vi "Micro-PL v10.5.0.vi"() -> ()   [LabVIEW 2010]
uses:
  drivers/Oxford ITC/ITCAPPS.LLB/ITCSetup.ctl
  drivers/Oxford ITC/ITCSUBS.LLB/ITCIO.ctl
  drivers/Oxford ITC/BUSGEN.LLB/OxfordAddress.ctl
  drivers/Oxford ITC/ITCSUBS.LLB/ITCVersion.ctl
  subvi/ESA-C/TypeDefs/ESA-C Live Controls v10.4.0.ctl
  subvi/ESA-C/TypeDefs/ESA-C Current Values.ctl
  subvi/ESA-C/TypeDefs/ESA-C Connection Settings.ctl
  subvi/ESA-C/TypeDefs/ESA-C Set Positions.ctl
  subvi/ITC503/TypeDefs/ITC503 Settings.ctl
  subvi/ITC503/TypeDefs/ITC503 Current Values.ctl
  subvi/iHR550/TypeDefs/iHR Current Values.ctl
  subvi/iHR550/TypeDefs/iHR Settings.ctl
  subvi/Mapping/TypeDefs/Mapping Spectra Params.ctl
  <vilib>/Utility/miscctls.llb/LVBoundsTypeDef.ctl
  subvi/Symphony/TypeDefs/Symphony Area Format.ctl
  <vilib>/Utility/miscctls.llb/LVPointTypeDef.ctl
  subvi/Mapping/TypeDefs/Mapping Input Parameters.ctl
  subvi/Global Variables.vi
  <vilib>/Analysis/NI_AALBase.lvlib
panel:
  out "Spectrum Raw PX":dbl[][](array[numeric])
  out "Image Raw":i32[][](array[numeric])
  in  "Wavelength Recalculate":bool
  out "CCD Error":errorcluster
  out "Firmware":string="V1.20 CCD_4000"
  out "CCD Gain Number":i32[](array[numeric])=[10, 11, 12, 13, 8, 2]
  out "CCD ADC Number":i32[](array[numeric])=[0, 1, 2, 3, 4]
  out "JYCCDLib.IJYCCDReqd":refnum<k7>
  out "Spectrum Raw WL":dbl[][](array[numeric])
  out "Mapping State Storage":bool
  out "Drive Copy Target":bool
  in  "CCD Shutter":bool caption="Shutter:"
  out "Measurement Running":bool
  out "ITC Running":bool
  out "Drive Running":bool
  out "CCD Running":bool
  out "Mono Running":bool
  in  "Exit":bool
  out "Mono Status":bool
  out "Drive Status":bool
  out "CCD Status":bool
  out "ITC Status":bool
  in  "Register":enum32{"Devices", "Acquisition / Mapping"}(tab)
  in  "CCD Gain":u16(ring)=1 caption="Gain Mode" items=["High Light", "Best Dynamic Range", "High Sensitivity"]
  in  "Image Mode":bool caption="Image Mode?"
  in  "CCD Names":u16(ring) caption="CCD ID" items=["Symphony II"]
  in  "CCD Connect":bool
  out "CCD Temperature":dbl caption="Temp. (°C)" min=10.0 max=160.0 step=0.1 format="%.1f"
  out "CCD Pixel X":i32=2048 caption="X Pixels"
  out "CCD Pixel Y":i32=512 caption="Y Pixels"
  out "CCD Data Size":i32=2048 caption="Data Size"
  in  "CCD ADC":u16(ring) caption="ADC Frequency" items=["20 kHz       ", " 1 MHz       ", " 1 MHz Ultra ", "500 kHz Wrap"]
  in  "CCD Configure":bool
  in  "CCD Area":T1={"XStart"=1, "YStart"=1, "XStop"=2048, "YStop"=512, "XBin"=1, "YBin"=1}
  in  "Snapshot Folder":path=path "C:/Users/WET-KORR/Desktop/Screenshots"
  in  "Camera Name":string="HD USB Camera"
  out "CCD Temp Graph":dbl(graph)=-134.538067
  out "CCD IDs":u16(ring) items=["CCD1"]
  out "ITC Current Values":T2 {"ITC503 Gradient" format="%.2f"; "ITC503 Setpoint" min=-273.0 max=300000.0 step=0.0001 format="%.1f"; "ITC503 I" format="%_1f"; "ITC503 P" format="%_1f"; "ITC503 Temperature" min=0.0 max=1645.0 step=1e-05 format="%.2f"; "ITC503 Heater" min=0.0 max=100.0 step=0.01 scale=0.0..100.0}
  in  "ITC Settings":T3={"ITC503 Set Setpoint"=0.0, "ITC503 Set Auto Heater"=TRUE, "ITC503 Set Auto PID"=TRUE, "P"=0.0, "I"=0.0, "D"=0.0} {"D" min=0.0 max=100.0 step=0.1 format="%.1f"; "I" min=0.0 max=100.0 step=0.1 format="%.1f"; "P" min=0.0 max=100.0 step=0.1 format="%.1f"; "ITC503 Set Setpoint" min=-273.0 max=300000.0 step=0.1 format="%.1f"}
  in  "ITC Configure":bool
  in  "ITC Connect":bool
  in  "ITC Selector":u16(ring) caption="Select Device" items=["ITC503s"]
  out "Drive Current Values":T4 {"Position"."Drive Z Position" min=-273.0 max=300000.0 step=0.0001 format="%.1f"; "Position"."Drive Y Position" min=-273.0 max=300000.0 step=0.0001 format="%.1f"; "Position"."Drive X Position" min=-273.0 max=300000.0 step=0.0001 format="%.1f"; "Voltages"."Drive Z Voltage" min=-273.0 max=300000.0 step=0.0001 format="%.1f"; "Voltages"."Drive Y Voltage" min=-273.0 max=300000.0 step=0.0001 format="%.1f"; "Voltages"."Drive X Voltage" min=-273.0 max=300000.0 step=0.0001 format="%.1f"}
  in  "Drive Connection":T5={"Objective GPIB-Port"=4, "Stage GPIB-Port"=4, "Drive Selector"=0, "Drive Velocity (V/s)"=5.0} {"Drive Velocity (V/s)" min=10.0 max=160.0 step=0.1 format="%.1f"; "Drive Selector" items=["Obj.", "Stage"]; "Stage GPIB-Port" min=1 max=20 step=1 format="%#.0f"; "Objective GPIB-Port" min=1 max=20 step=1 format="%#.0f"}
  in  "Drive Connect":bool
  in  "Mono Force Init":bool=TRUE caption="iHR550 Force Init"
  in  "Mono Connect":bool
  in  "Mono ID":string(combo)="iHR550" caption="Monochromator ID"
  out "Mono Timing":u32 caption="Mono"
  out "Drive Timing":u32 caption="Drive"
  out "ITC Timing":u32 caption="ITC"
  out "CCD Timing":u32 caption="CCD"
  in  "Spectrum Axis":u16(ring)=1 caption="Axis" items=["Pixel", "Wavelength", "Energy"]
  in  "Spectrum Autosave":bool caption="iHR550 Force Init"
  in  "CCD Preview":bool
  in  "CCD Acquire":bool
  in  "Spectrum Settings":T6={"Integration Time"=1.0, "Repetitions"=1, "Mapping Spectra"=TRUE} caption="Mapping Spectra Settings" {"Repetitions" min=1 max=100 step=1; "Integration Time" min=0.1 max=6000.0 step=0.1 format="%.1f"}
  in  "CCD Current Rep.":string="0/0"
  out "Spectrum":cluster{dbl[], dbl[]}[](graph)
  out "Image":dbl[][](graph)
  in  "Spectrum Noise":i64 caption="Noise Level"
  in  "Spectrum Load":bool
  in  "Spectrum Save":bool
  in  "Spectrum Maximize":bool
  in  "Video Show":bool
  in  "Drive GoTo":bool caption="Objective Move Abs."
  in  "Drive New Positions":T7 {"Drive X Set" min=10.0 max=160.0 step=0.1 format="%.1f"; "Drive Z Set" min=10.0 max=160.0 step=0.1 format="%.1f"; "Drive Y Set" min=10.0 max=160.0 step=0.1 format="%.1f"}
  in  "Mapping Start":bool
  in  "Mono Configure":bool
  in  "Mono Settings":T8={"iHR550 Set Exit Mirror"=2, "iHR550 Set Side Exit"=0.0, "iHR550 Set Front Entrance"=0.0, "iHR550 Set Wavelength"=897.9988, "iHR550 Set Grating"=0, "iHR550 Set Grating Switch"=FALSE, "iHR550 Set Wavelength Switch"=FALSE, "iHR550 Set Mirror Switch"=FALSE, "iHR550 Set Slits Switch"=FALSE} {"iHR550 Set Grating" items=["1800"=1, "600"=2, "150"=3]; "iHR550 Set Wavelength" min=0.0 max=1500.0 step=1.0; "iHR550 Set Side Exit" min=0.0 max=2000.0 step=1.0; "iHR550 Set Exit Mirror" items=["Front"=2, "Side"=3]}
  out "Mono Current Values":T9={"iHR 550 Front Entrance"=0.0, "iHR550 Side Exit"=0.0, "iHR550 Wavelength"=897.9988, "iHR550 Exit Mirror"=2, "iHR550 Grating"="1", "Grating Index"=1} {"iHR550 Exit Mirror" items=["EntranceMirror", "ExitMirror", "Front", "Side"]}
  out "Drive Live Current Values":T4 {"Position"."Drive Z Position" min=-273.0 max=300000.0 step=0.0001 format="%.1f"; "Position"."Drive Y Position" min=-273.0 max=300000.0 step=0.0001 format="%.1f"; "Position"."Drive X Position" min=-273.0 max=300000.0 step=0.0001 format="%.1f"; "Voltages"."Drive Z Voltage" min=-273.0 max=300000.0 step=0.0001 format="%.1f"; "Voltages"."Drive Y Voltage" min=-273.0 max=300000.0 step=0.0001 format="%.1f"; "Voltages"."Drive X Voltage" min=-273.0 max=300000.0 step=0.0001 format="%.1f"}
  in  "Drive Live Controls":T10={"Move Step"=1.0, "Move Home"=FALSE, "Move Down"=FALSE, "Move Up"=FALSE, "Move Left"=FALSE, "Move Right"=FALSE, "Move Out"=FALSE, "Move In"=FALSE} {"Move Step" min=0.0 max=30.0 step=0.1 format="%.1f"}
  out "ITC Temp Storage":dbl
  out "Runtime":u32
  out "ITC Gradient Time":i64
  out "ITC Read":bool
  out "CCD Read":bool
  out "Mono Read":bool
  out "Drive Read":bool
  out "Spectrum Properties":cluster{"Position":T11, "Plot Area Size":T11}={"Position"={"Width"=36, "Height"=367}, "Plot Area Size"={"Width"=496, "Height"=264}}
  in  "Auto Folder":path caption="Ausgewählter Pfad"
  out "Wavelengths (nm)":dbl[](array[numeric])
  out "iHR550 RefNum":refnum<k7> caption="Mono RefNum out"
  out "ITC Setup":T12={"Description"="", "IO Info"={"Address"={"Com Port"=1, "ISOBUS Address"=1, "GPIB Address"=24, "Communication"=enum."ISOBUS"}, "Version"=enum."ITC503", "Ch 1 dec places"=1, "Ch 2 dec places"=1, "Ch 3 dec places"=1, "Ch1 Name"="", "Ch2 Name"="", "Ch3 Name"=""}}
  # "Correlation Setup"
  # "Active"
  # "Active"
  # "ITC"
  # "iHR"
  # "Drive"
  # "CCD"
  # "Status"
  # "CCD"
  # "ITC"
  # "iHR"
  # "Drive"
  # "CCD"
  # "Video"
  # "Cryostat"
  # "Drives"
  # "Monochromator"
  # "Timing"
  # "Drive Control"
  # "CCD"
  # "Acquisition"
  # "Mapping"
  # "Launch the Spectral Mapping VI and Raman Tool Set 2.0 in a new window."
  # "Monochromator"
  # "XY"
  # "Z"
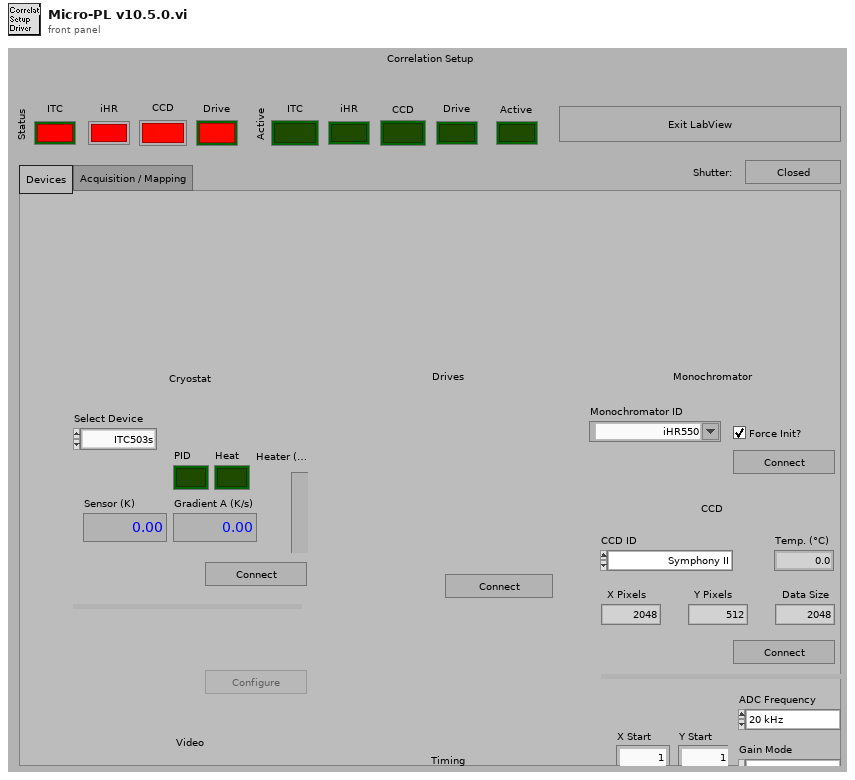
[diagram p1: front panel]
types:
  T1 = typedef "Symphony Area Format.ctl" = cluster{"XStart":i32, "YStart":i32, "XStop":i32, "YStop":i32, "XBin":i32, "YBin":i32}
  T2 = typedef "ITC503 Current Values.ctl" = cluster{"ITC503 Heater":dbl, "ITC503 Temperature":dbl, "ITC503 P":dbl, "ITC503 I":dbl, "ITC503 D":dbl, "ITC503 Setpoint":dbl, "ITC503 Gradient":dbl, "ITC503 Heater Auto":bool, "ITC503 PID Auto":bool}
  T3 = typedef "ITC503 Settings.ctl" = cluster{"ITC503 Set Setpoint":dbl, "ITC503 Set Auto Heater":bool, "ITC503 Set Auto PID":bool, "P":dbl, "I":dbl, "D":dbl}
  T4 = typedef "ESA-C Current Values.ctl" = cluster{"Voltages":cluster{"Drive X Voltage":dbl, "Drive Y Voltage":dbl, "Drive Z Voltage":dbl}, "Position":cluster{"Drive X Position":dbl, "Drive Y Position":dbl, "Drive Z Position":dbl}}
  T5 = typedef "ESA-C Connection Settings.ctl" = cluster{"Objective GPIB-Port":i32, "Stage GPIB-Port":i32, "Drive Selector":u16, "Drive Velocity (V/s)":dbl}
  T6 = typedef "Mapping Spectra Params.ctl" = cluster{"Integration Time":dbl, "Repetitions":u16, "Mapping Spectra":bool}
  T7 = typedef "ESA-C Set Positions.ctl" = cluster{"Drive X Set":dbl, "Drive Y Set":dbl, "Drive Z Set":dbl}
  T8 = typedef "iHR Settings.ctl" = cluster{"iHR550 Set Exit Mirror":u16, "iHR550 Set Side Exit":dbl, "iHR550 Set Front Entrance":dbl, "iHR550 Set Wavelength":dbl, "iHR550 Set Grating":u16, "iHR550 Set Grating Switch":bool, "iHR550 Set Wavelength Switch":bool, "iHR550 Set Mirror Switch":bool, "iHR550 Set Slits Switch":bool}
  T9 = typedef "iHR Current Values.ctl" = cluster{"iHR 550 Front Entrance":dbl, "iHR550 Side Exit":dbl, "iHR550 Wavelength":dbl, "iHR550 Exit Mirror":i32, "iHR550 Grating":string, "Grating Index":i32}
  T10 = typedef "ESA-C Live Controls v10.4.0.ctl" = cluster{"Move Step":dbl, "Move Home":bool, "Move Down":bool, "Move Up":bool, "Move Left":bool, "Move Right":bool, "Move Out":bool, "Move In":bool}
  T11 = typedef "LVBoundsTypeDef.ctl" = cluster{"Width":u32, "Height":u32}
  T12 = typedef "ITCSetup.ctl" = cluster{"Description":string, "IO Info":T13}
  T13 = typedef "ITCIO.ctl" = cluster{"Address":T14, "Version":T15, "Ch 1 dec places":i16, "Ch 2 dec places":i16, "Ch 3 dec places":i16, "Ch1 Name":string, "Ch2 Name":string, "Ch3 Name":string}
  T14 = typedef "OxfordAddress.ctl" = cluster{"Com Port":i32, "ISOBUS Address":i32, "GPIB Address":i16, "Communication":enum16{"RS232", "ISOBUS", "GPIB", "Gateway"}}
  T15 = typedef "ITCVersion.ctl" = enum16{"ITC502", "ITC503", "ITC601"}
  T16 = enum8{"Enabled", "Disabled", "Disabled and Grayed Out"}
  T17 = typedef "LVPointTypeDef.ctl" = cluster{"Horizontal":i16, "Vertical":i16}
  T18 = typedef "Mapping Input Parameters.ctl" = cluster{"Drive Connection Settings":T5, "ITC503 Current Values":T2, "Wavelengths (nm)":dbl[], "Drive Current Values":T4, "iHR Current Values":T9, "Spectra Settings":T6, "CCD3500 Temperature":dbl, "Simulate Drive":bool, "Simulate Spectra":bool, "JYCCDLib.IJYCCDReqd":refnum<k7>}
  T19 = cluster{"Intensities":dbl[], "Wavelengths":dbl[]}[]
  T20 = cluster{"Drive X Position":dbl, "Drive Y Position":dbl, "Drive Z Position":dbl}
  T21 = typedef "LVPositionTypeDef.ctl" = cluster{"Left":i32, "Top":i32}
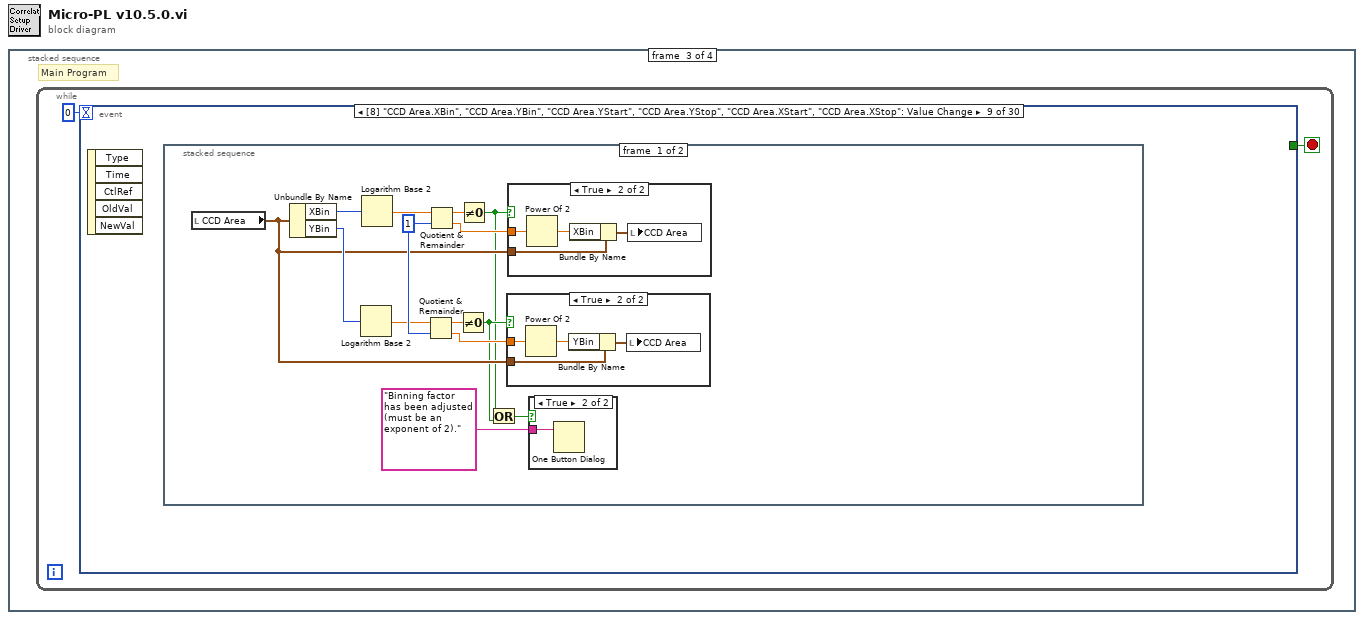
[diagram p0: block diagram]
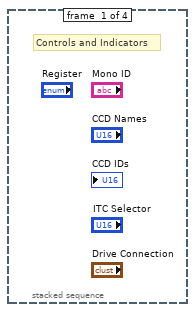
[diagram p2: hidden frame]
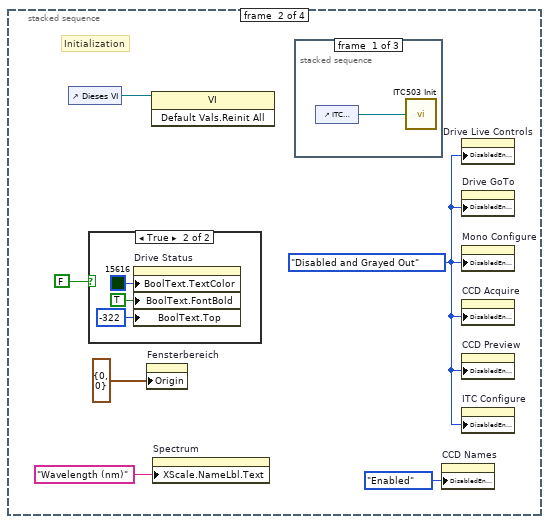
[diagram p3: hidden frame]
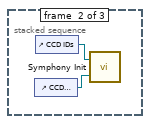
[diagram p4: hidden frame]
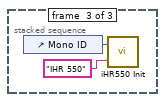
[diagram p5: hidden frame]
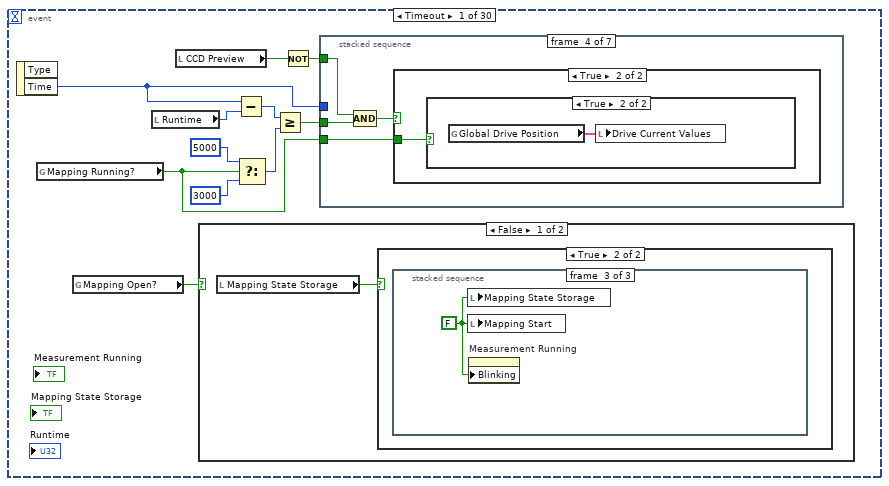
[diagram p7: hidden frame]
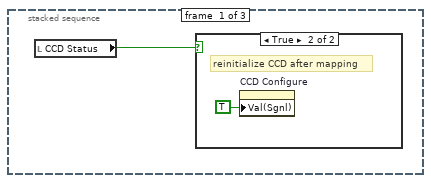
[diagram p9: hidden frame]
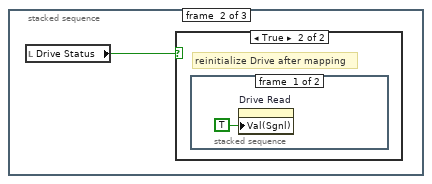
[diagram p11: hidden frame]
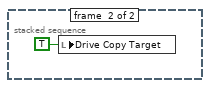
[diagram p13: hidden frame]
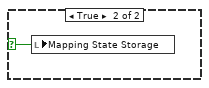
[diagram p14: hidden frame]
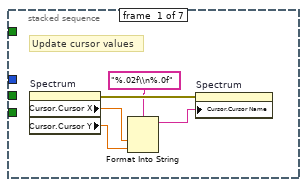
[diagram p15: hidden frame]
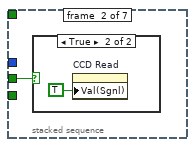
[diagram p16: hidden frame]
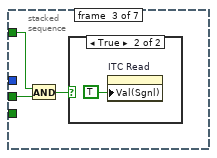
[diagram p18: hidden frame]
diagram:
  n1 = stacked-sequence {
    frame #0 {
      # "Controls and Indicators"
    }
    frame #1 {
      w3 = T16."Disabled and Grayed Out" ("Deaktiviert")
      # "Initialization"
      n2 = control-ref of="Dieses VI"() -> (w6:refnum<vi>)
      n3 = case shown="True" FALSE {
        frame False {
        }
        frame True {
          n4 = property on="Drive Status" class="Bool (strict)"("BoolText.TextColor"=u32 15616, "BoolText.FontBold"=TRUE ("Boolescher Text.Schriftart:Fett"), "BoolText.Top"=-322 ("Boolescher Text.Position:Oben")) -> ()  [unwired: 2 in, 2 out]
        }
      }
      n5 = property on="Fensterbereich" class="Pane"("Origin"=T17 {"Horizontal"=0, "Vertical"=0}) -> ()  [unwired: 2 in, 2 out]
      n6 = invoke class="VI" method="Default Vals.Reinit All"(reference=w6) -> ()  [unwired: 2 in, 3 out]
      n7 = property on="Spectrum" class="XYGraph (strict)"("XScale.NameLbl.Text"="Wavelength (nm)" ("X Scale.Name Label.Text")) -> ()  [unwired: 2 in, 2 out]
      n8 = stacked-sequence {
        frame #0 {
          n9 = control-ref of="ITC Selector"() -> (w7:refnum<vi>)
          n10 = call "ITC503 Init.vi"("ITC Selector"=w7) -> ()  [unwired: 1 in]
        }
        frame #1 {
          n11 = control-ref of="CCD Names"() -> (w8:refnum<vi>)
          n12 = control-ref of="CCD IDs"() -> (w9:refnum<vi>)
          n13 = call "Symphony Init.vi"("Device Names"=w8, "Device IDs"=w9) -> ()
        }
        frame #2 {
          n14 = control-ref of="Mono ID"() -> (w11:refnum<vi>)
          n15 = call "iHR550 Init.vi"("Mono ID"=w11, "Target ID"="IHR 550") -> ()  [unwired: 1 in]
        }
      }
      n16 = property on="CCD Names" class="Ring (strict)"("DisabledEnum"=T16."Enabled" ("Disabled")) -> ()  [unwired: 2 in, 2 out]
      n17 = property on="Drive Live Controls" class="Clust (strict)"("DisabledEnum"=w3) -> ()  [unwired: 2 in, 2 out]
      n18 = property on="Drive GoTo" class="Bool (strict)"("DisabledEnum"=w3) -> ()  [unwired: 2 in, 2 out]
      n19 = property on="Mono Configure" class="Bool (strict)"("DisabledEnum"=w3) -> ()  [unwired: 2 in, 2 out]
      n20 = property on="CCD Acquire" class="Bool (strict)"("DisabledEnum"=w3) -> ()  [unwired: 2 in, 2 out]
      n21 = property on="CCD Preview" class="Bool (strict)"("DisabledEnum"=w3) -> ()  [unwired: 2 in, 2 out]
      n22 = property on="ITC Configure" class="Bool (strict)"("DisabledEnum"=w3) -> ()  [unwired: 2 in, 2 out]
    }
    frame #2 {
      # "Main Program"
      n23 = while "Main-Program" {
        stop <- w16 stop-if-true
        n24 = event shown="[8] \"CCD Area.XBin\", \"CCD Area.YBin\", \"CCD Area.YStart\", \"CCD Area.YStop\", \"CCD Area.XStart\", \"CCD Area.XStop\": Value Change" {
          selector: _ -> [_ _ _ _ _ _ _ _ _ _ _ _ _ _ _ _ _ _ _ _ _ _ _ _ _ _ _ _ _ _]
          dyn-events: _ -> [_ _ _ _ _ _ _ _ _ _ _ _ _ _ _ _ _ _ _ _ _ _ _ _ _ _ _ _ _ _]
          timeout: 0 -> [_ _ _ _ _ _ _ _ _ _ _ _ _ _ _ _ _ _ _ _ _ _ _ _ _ _ _ _ _ _]
          tunnel: [_ w64 _ _ _ _ _ _ _ _ _ _ _ _ _ _ _ _ _ _ _ _ _ _ _ _ _ _ _ _] -> w16
          event Timeout {
            n25 = event-data() -> ("Time"=w23:u32)  [unwired: 1 in, 1 out]
            n26 = global read "Global Variables.vi" "Mapping Running?"() -> (w18:bool)
            n27 = global read "Global Variables.vi" "Mapping Open?"() -> (w17:bool)
            n28 = local read "Runtime"() -> (w22:u32)
            n29 = local read "CCD Preview"() -> (w25:bool)
            n30 = case shown="False" w17 {
              selector: w17 -> [_ w35]
              frame False {
                n31 = local read "Mapping State Storage"() -> (w28:bool)
                n32 = case shown="True" w28 {
                  frame False {
                  }
                  frame True {
                    n33 = stacked-sequence {
                      frame #0 {
                        n34 = local read "CCD Status"() -> (w29:bool)
                        n35 = case shown="True" w29 {
                          frame False {
                          }
                          frame True {
                            # "reinitialize CCD after mapping"
                            n36 = property on="CCD Configure" class="Bool (strict)"("Val(Sgnl)"=TRUE ("Value (Signaling)")) -> ()  [unwired: 2 in, 2 out]
                          }
                        }
                      }
                      frame #1 {
                        n37 = local read "Drive Status"() -> (w31:bool)
                        n38 = case shown="True" w31 {
                          frame False {
                          }
                          frame True {
                            # "reinitialize Drive after mapping"
                            n39 = stacked-sequence {
                              frame #0 {
                                n40 = property on="Drive Read" class="Bool (strict)"("Val(Sgnl)"=TRUE ("Value (Signaling)")) -> ()  [unwired: 2 in, 2 out]
                              }
                              frame #1 {
                                n41 = local write "Drive Copy Target"(TRUE ("Copy Drive Target")) -> ()
                              }
                            }
                          }
                        }
                      }
                      frame #2 {
                        w34 = FALSE ("Mapping Start")
                        n42 = local write "Mapping State Storage"(w34) -> ()
                        n43 = local write "Mapping Start"(w34) -> ()
                        n44 = property on="Measurement Running" class="Bool (strict)"("Blinking"=w34) -> ()  [unwired: 2 in, 2 out]
                      }
                    }
                  }
                }
              }
              frame True {
                n45 = local write "Mapping State Storage"(w35) -> ()
              }
            }
            n46 = Subtract(x=w23, y=w22) -> (x-y=w26:u32)
            n47 = Select(t=u32 5000 ("y"), s=w18, f=u32 3000 ("y")) -> (s? t:f=w19:u32)
            n48 = Greater Or Equal?(x=w26, y=w19) -> (x >= y?=w27:bool)
            n49 = Not(x=w25) -> (.not. x?=w24:bool)
            n50 = stacked-sequence {
              tunnel: w27 -> [_ w41 w45 w50 w57 _ w61]
              tunnel: w23 -> [_ _ _ _ _ _ w62]
              tunnel: w24 -> [_ _ w44 w49 w56 w59 _]
              tunnel: w18 -> [_ _ _ w47 w54 _ _]
              frame #0 {
                # "Update cursor values"
                n51 = property on="Spectrum" class="XYGraph (strict)"() -> (error out=w40:errorcluster, "Cursor.Cursor X"=w39:dbl, "Cursor.Cursor Y"=w38:dbl)  [unwired: 2 in, 1 out]
                n52 = Format Into String(format string="%.02f\\n%.0f", w39, w38) -> (resulting string=w36:string)  [unwired: 2 in, 1 out]
                n53 = property on="Spectrum" class="XYGraph (strict)"(error in=w40, "Cursor.Cursor Name"=w36) -> ()  [unwired: 1 in, 2 out]
              }
              frame #1 {
                n54 = case shown="True" w41 {
                  frame False {
                  }
                  frame True {
                    n55 = property on="CCD Read" class="Bool (strict)"("Val(Sgnl)"=TRUE ("Value (Signaling)")) -> ()  [unwired: 2 in, 2 out]
                  }
                }
              }
              frame #2 {
                n56 = And(x=w44, y=w45) -> (x .and. y?=w43:bool)
                n57 = case shown="True" w43 {
                  frame False {
                  }
                  frame True {
                    n58 = property on="ITC Read" class="Bool (strict)"("Val(Sgnl)"=TRUE ("Value (Signaling)")) -> ()  [unwired: 2 in, 2 out]
                  }
                }
              }
              frame #3 {
                n59 = Compound Arithmetic op=AND(w49, w50) -> (w48:bool)
                n60 = case shown="True" w48 {
                  tunnel: w47 -> [_ w51]
                  frame False {
                  }
                  frame True {
                    n61 = case shown="True" w51 {
                      frame False {
                        n62 = property on="Drive Read" class="Bool (strict)"("Val(Sgnl)"=TRUE ("Value (Signaling)")) -> ()  [unwired: 2 in, 2 out]
                      }
                      frame True {
                        n63 = global read "Global Variables.vi" "Global Drive Position"() -> (w53:T4)
                        n64 = local write "Drive Current Values"(w53) -> ()
                      }
                    }
                  }
                }
              }
              frame #4 {
                n65 = Compound Arithmetic op=AND(w56, w57, w54) -> (w55:bool)
                n66 = case shown="True" w55 {
                  frame False {
                  }
                  frame True {
                    n67 = property on="Mono Read" class="Bool (strict)"("Val(Sgnl)"=TRUE ("Value (Signaling)")) -> ()  [unwired: 2 in, 2 out]
                  }
                }
              }
              frame #5 {
                n68 = case shown="False" w59 {
                  frame False {
                    n69 = property on="CCD Acquire" class="Bool (strict)"("Val(Sgnl)"=TRUE ("Wert (signalisierend)")) -> ()  [unwired: 2 in, 2 out]
                  }
                  frame True {
                  }
                }
              }
              frame #6 {
                # "Set runtime counter"
                n70 = case shown="True" w61 {
                  tunnel: w62 -> [_ w63]
                  frame False {
                  }
                  frame True {
                    n71 = local write "Runtime"(w63) -> ()
                  }
                }
              }
            }
          }
          event "Exit": Value Change {
            n72 = event-data() -> ("NewVal"=w64:bool)  [unwired: 1 in, 4 out]
            n73 = stacked-sequence {
              frame #0 {
                n74 = local read "CCD Status"() -> (w65:bool)
                n75 = case shown="True" w65 {
                  frame False {
                  }
                  frame True {
                    n76 = property on="CCD Connect" class="Bool (strict)"("Val(Sgnl)"=FALSE ("Value (Signaling)")) -> ()  [unwired: 2 in, 2 out]
                  }
                }
              }
              frame #1 {
                n77 = local read "Mono Status"() -> (w67:bool)
                n78 = case shown="True" w67 {
                  frame False {
                  }
                  frame True {
                    n79 = property on="Mono Connect" class="Bool (strict)"("Val(Sgnl)"=FALSE ("Value (Signaling)")) -> ()  [unwired: 2 in, 2 out]
                  }
                }
              }
              frame #2 {
                n80 = local read "ITC Status"() -> (w69:bool)
                n81 = case shown="True" w69 {
                  frame False {
                  }
                  frame True {
                    n82 = property on="ITC Connect" class="Bool (strict)"("Val(Sgnl)"=FALSE ("Value (Signaling)")) -> ()  [unwired: 2 in, 2 out]
                  }
                }
              }
              frame #3 {
                n83 = local read "Drive Status"() -> (w71:bool)
                n84 = case shown="True" w71 {
                  frame False {
                  }
                  frame True {
                    n85 = property on="Drive Status" class="Bool (strict)"("Val(Sgnl)"=FALSE ("Value (Signaling)")) -> ()  [unwired: 2 in, 2 out]
                  }
                }
              }
            }
          }
          event "Mono Connect": Value Change {
            n86 = event-data() -> ("NewVal"=w73:bool)  [unwired: 1 in, 4 out]
            n87 = stacked-sequence {
              tunnel: w73 -> [_ w76 _]
              frame #0 {
                n88 = property on="Mono Running" class="Bool (strict)"("Blinking"=TRUE ("Blinkend")) -> ()  [unwired: 2 in, 2 out]
              }
              frame #1 {
                n89 = case shown="False" w76 {
                  selector: w76 -> [w80 _]
                  tunnel: [w80 w92] -> w75
                  frame False {
                    # "disconnect"
                  }
                  frame True {
                    # "connect"
                    n90 = local read "Mono Force Init"() -> (w90:bool)
                    n91 = control-ref of="iHR550 Set Grating"() -> (w91:refnum<vi>)
                    n92 = local read "Mono ID"() -> (w93:string)
                    n93 = call "iHR550 Connect.vi"("Force\nInitialization"=w90, "Grating Selector"=w91, "Mono ID"=w93) -> ("Initialized"=w92:bool, "iHR550 RefNum"=w89:refnum<k7>)  [unwired: 2 in, 4 out]
                    n94 = local write "iHR550 RefNum"(w89) -> ()
                    n95 = call "iHR550 Read Values v10.5.0.vi"("JYMONOLib.IJYMonoReqd"=w89) -> ("iHR Current Values"=w81:T9)  [unwired: 1 in]
                    n96 = Unbundle By Name(w81) -> ("iHR 550 Front Entrance"=w87:dbl, "iHR550 Side Exit"=w86:dbl, "iHR550 Wavelength"=w85:dbl, "iHR550 Exit Mirror"=w84:i32, "Grating Index"=w82:i32)
                    n97 = local write "Mono Current Values"(w81) -> ()
                    n98 = Bundle By Name(cluster=T8 {"iHR550 Set Exit Mirror"=0, "iHR550 Set Side Exit"=0.0, "iHR550 Set Front Entrance"=0.0, "iHR550 Set Wavelength"=0.0, "iHR550 Set Grating"=0, "iHR550 Set Grating Switch"=FALSE, "iHR550 Set Wavelength Switch"=FALSE, "iHR550 Set Mirror Switch"=FALSE, "iHR550 Set Slits Switch"=FALSE} ("iHR Settings"), "iHR550 Set Front Entrance"=w87, "iHR550 Set Side Exit"=w86, "iHR550 Set Wavelength"=w85, "iHR550 Set Exit Mirror"=w84, "iHR550 Set Grating"=w82) -> (w83:T8)
                    n99 = local write "Mono Settings"(w83) -> ()
                  }
                }
                n100 = case shown="False" w75 {
                  tunnel: [T16."Disabled and Grayed Out" ("Deaktiviert") T16."Enabled" ("Deaktiviert")] -> w77
                  frame False {
                  }
                  frame True {
                  }
                }
                n101 = local write "Mono Connect"(w75) -> ()
                n102 = local write "Mono Status"(w75) -> ()
                n103 = property on="Mono Configure" class="Bool (strict)"("DisabledEnum"=w77) -> ()  [unwired: 2 in, 2 out]
              }
              frame #2 {
                w95 = TRUE ("Wert (signalisierend)")
                w94 = FALSE ("Blinkend")
                n104 = local write "Mono Force Init"(w94) -> ()
                n105 = property on="Mono Running" class="Bool (strict)"("Blinking"=w94) -> ()  [unwired: 2 in, 2 out]
                n106 = property on="Mono Read" class="Bool (strict)"("Val(Sgnl)"=w95) -> ()  [unwired: 2 in, 2 out]
                n107 = property on="Wavelength Recalculate" class="Bool (strict)"("Val(Sgnl)"=w95) -> ()  [unwired: 2 in, 2 out]
              }
            }
          }
          event "Mono Read": Value Change {
            n108 = event-data() -> ("NewVal"=w99:bool)  [unwired: 1 in, 4 out]
            n109 = local read "Mono Status"() -> (w98:bool)
            n110 = And(x=w98, y=w99) -> (x .and. y?=w97:bool)
            n111 = case shown="True" w97 {
              tunnel: [u32 0 w101] -> w96
              frame False {
              }
              frame True {
                n112 = stacked-sequence {
                  seq-local: [w102 _ _] -> [_ _ w105]
                  tunnel: [_ _ w106] -> w101
                  frame #0 {
                    n113 = Tick Count (ms)() -> (millisecond timer value=w102:u32)
                  }
                  frame #1 {
                    n114 = local read "iHR550 RefNum"() -> (w104:refnum<k7>)
                    n115 = call "iHR550 Read Values v10.5.0.vi"("JYMONOLib.IJYMonoReqd"=w104) -> ("iHR Current Values"=w103:T9)  [unwired: 1 in]
                    n116 = local write "Mono Current Values"(w103) -> ()
                    n117 = global write "Global Variables.vi" "Global iHR Values"(w103) -> ()
                  }
                  frame #2 {
                    n118 = Tick Count (ms)() -> (millisecond timer value=w107:u32)
                    n119 = Subtract(x=w107, y=w105) -> (x-y=w106:u32)
                  }
                }
              }
            }
            "Mono Timing" <- w96
          }
          event "Mono Configure": Value Change {
            n120 = event-data() -> ("NewVal"=w108:bool)  [unwired: 1 in, 4 out]
            n121 = stacked-sequence {
              tunnel: w108 -> [_ w110 _]
              frame #0 {
                n122 = property on="Mono Running" class="Bool (strict)"("Blinking"=TRUE ("Blinkend")) -> ()  [unwired: 2 in, 2 out]
              }
              frame #1 {
                n123 = local read "Mono Status"() -> (w112:bool)
                n124 = And(x=w112, y=w110) -> (x .and. y?=w111:bool)
                n125 = case shown="True" w111 {
                  frame False {
                  }
                  frame True {
                    n126 = stacked-sequence {
                      frame #0 {
                        w116 = u16 2 items=["Front"=2, "Side"=3] ("Entrance Mirror")
                        n127 = local read "iHR550 RefNum"() -> (w113:refnum<k7>)
                        n128 = local read "Mono Settings"() -> (w114:T8)
                        n129 = call "iHR550 Set Values v10.5.0.vi"("Refnum out"=w113, "Entrance Mirror"=w116, "Target\nSide Entrance"=0.0 ("Target\nSide Entrance"), "iHR Settings"=w114) -> ()  [unwired: 11 in, 1 out]
                      }
                      frame #1 {
                        n130 = property on="Mono Read" class="Bool (strict)"("Val(Sgnl)"=TRUE ("Value (Signaling)")) -> ()  [unwired: 2 in, 2 out]
                      }
                      frame #2 {
                        n131 = property on="Wavelength Recalculate" class="Bool (strict)"("Val(Sgnl)"=TRUE ("Value (Signaling)")) -> ()  [unwired: 2 in, 2 out]
                      }
                    }
                  }
                }
              }
              frame #2 {
                w120 = FALSE ("Blinkend")
                n132 = property on="Mono Read" class="Bool (strict)"("Val(Sgnl)"=TRUE ("Wert (signalisierend)")) -> ()  [unwired: 2 in, 2 out]
                n133 = property on="Mono Running" class="Bool (strict)"("Blinking"=w120) -> ()  [unwired: 2 in, 2 out]
                n134 = local write "Mono Configure"(w120) -> ()
              }
            }
          }
          event "CCD Connect": Value Change {
            n135 = event-data() -> ("NewVal"=w121:bool)  [unwired: 1 in, 4 out]
            n136 = stacked-sequence {
              tunnel: w121 -> [_ w125 _]
              frame #0 {
                n137 = local read "CCD Names"() -> (w122:u16)
                n138 = property on="CCD Running" class="Bool (strict)"("Blinking"=TRUE ("Blinkend")) -> ()  [unwired: 2 in, 2 out]
                n139 = local write "CCD IDs"(w122) -> ()
              }
              frame #1 {
                n140 = case shown="True" w125 {
                  selector: w125 -> [w134 _]
                  tunnel: [w134 w143] -> w127
                  frame False {
                    # "disconnect"
                    n141 = local read "JYCCDLib.IJYCCDReqd"() -> (w133:refnum<k7>)
                    n142 = local read "CCD Error"() -> (w132:errorcluster)
                    n143 = Close Reference(reference=w133, error in (no error)=w132) -> ()  [unwired: 1 out]
                  }
                  frame True {
                    # "connect"
                    n144 = local read "CCD IDs"() -> (w148:u16)
                    n145 = property on="CCD IDs" class="Ring (strict)"() -> ("Chaînes []"=w147:string[])  [unwired: 2 in, 2 out]
                    n146 = Index Array(array=w147, index=w148) -> (element=w149:string)
                    n147 = call "Initialize CCD.vi"("Unique id:"=w149) -> ("activeYPixels"=w136:i32, "JYCCDLib.IJYCCDReqd"=w150:refnum<k7>, "activeXPixels"=w138:i32, "sortie d'erreur"=w151:errorcluster, "FirmwareVersion"=→"Firmware":string)  [unwired: 3 out]
                    "CCD Pixel X" <- w138
                    "CCD Pixel Y" <- w136
                    n148 = call "Trigger - Disable.vi"("Error In"=w151, "JYCCDLib.IJYCCDReqd"=w150) -> ("Error Out"=w145:errorcluster, "JYCCDLib.IJYCCDReqd"=w156:refnum<k7>)  [unwired: 4 out]
                    n149 = local read "CCD Area"() -> (w142:T1)
                    n150 = Bundle By Name(cluster=w142, "XStart"=1, "XStop"=w138, "YStart"=1, "YStop"=w136, "XBin"=1, "YBin"=1) -> (w141:T1)
                    n151 = local write "CCD Error"(w145) -> ()
                    n152 = call "Init ADC & Gain.vi"("JYCCDLib.IJYCCDReqd"=w156, "input error"=w145) -> ("ADC Number"=w152:i32[], "ADC description"=w154:string[], "Gain Number"=w153:i32[], "Gain description"=w155:string[])
                    n153 = local write "JYCCDLib.IJYCCDReqd"(w156) -> ()
                    n154 = local write "CCD Area"(w141) -> ()
                    n155 = local write "CCD ADC Number"(w152) -> ()
                    n156 = local write "CCD Gain Number"(w153) -> ()
                    n157 = property on="CCD ADC" class="Ring (strict)"("Chaînes []"=w154) -> ()  [unwired: 2 in, 2 out]
                    n158 = property on="CCD Gain" class="Ring (strict)"("Chaînes []"=w155) -> ()  [unwired: 2 in, 2 out]
                    n159 = call <vilib>:"Simple Error Handler.vi"("error in (no error)"=w145) -> ("error?"=w144:bool)  [unwired: 4 in, 4 out]
                    n160 = Not(x=w144) -> (.not. x?=w143:bool)
                  }
                }
                n161 = case shown="False" w127 {
                  tunnel: [T16."Disabled and Grayed Out" ("Deaktiviert") T16."Enabled" ("Deaktiviert")] -> w126
                  tunnel: [T16."Enabled" ("Deaktiviert") T16."Disabled and Grayed Out" ("Deaktiviert")] -> w124
                  frame False {
                  }
                  frame True {
                  }
                }
                n162 = property on="CCD Status" class="Bool (strict)"("BoolText.Visible"=w127) -> ()  [unwired: 2 in, 2 out]
                n163 = local write "CCD Connect"(w127) -> ()
                n164 = local write "CCD Status"(w127) -> ()
                n165 = property on="CCD Acquire" class="Bool (strict)"("DisabledEnum"=w126) -> ()  [unwired: 2 in, 2 out]
                n166 = property on="CCD Preview" class="Bool (strict)"("DisabledEnum"=w126) -> ()  [unwired: 2 in, 2 out]
                n167 = property on="CCD Names" class="Ring (strict)"("Désactivé"=w124) -> ()  [unwired: 2 in, 2 out]
                n168 = property on="CCD IDs" class="Ring (strict)"("Désactivé"=w124) -> ()  [unwired: 2 in, 2 out]
              }
              frame #2 {
                w157 = TRUE ("Wert (signalisierend)")
                n169 = property on="CCD Configure" class="Bool (strict)"("Val(Sgnl)"=w157) -> (error out=w158:errorcluster)  [unwired: 2 in, 1 out]
                n170 = property on="CCD Running" class="Bool (strict)"("Blinking"=FALSE ("Blinkend")) -> ()  [unwired: 2 in, 2 out]
                n171 = property on="CCD Read" class="Bool (strict)"(error in=w158, "Val(Sgnl)"=w157) -> ()  [unwired: 1 in, 2 out]
              }
            }
          }
          event "CCD Read": Value Change {
            n172 = event-data() -> ("NewVal"=w163:bool)  [unwired: 1 in, 4 out]
            n173 = local read "CCD Status"() -> (w162:bool)
            n174 = And(x=w162, y=w163) -> (x .and. y?=w161:bool)
            n175 = case shown="True" w161 {
              tunnel: [u32 0 w165] -> w160
              frame False {
              }
              frame True {
                n176 = stacked-sequence {
                  seq-local: [_ w167 _ _] -> [_ _ w172 _]
                  seq-local: [w166 _ _ _] -> [_ _ _ w183]
                  tunnel: [_ _ _ w184] -> w165
                  frame #0 {
                    n177 = Tick Count (ms)() -> (millisecond timer value=w166:u32)
                  }
                  frame #1 {
                    w168 = u16 0 items=["° Celsius", "Kelvin", "° Farenheit"] ("units")
                    n178 = local read "JYCCDLib.IJYCCDReqd"() -> (w171:refnum<k7>)
                    n179 = local read "CCD Error"() -> (w169:errorcluster)
                    n180 = call "read temperature.vi"("entrée d'erreur (pas d'erreur)"=w169, "units"=w168, "JYCCDLib.IJYCCDReqd"=w171) -> ("error out"=w170:errorcluster, "Current Temperature"=w167:dbl)
                    n181 = local write "CCD Temp Graph"(w167) -> ()
                    n182 = local write "CCD Error"(w170) -> ()
                    n183 = local write "CCD Temperature"(w167) -> ()
                  }
                  frame #2 {
                    n184 = Greater?(x=w172, y=-130.0) -> (0:w173:bool)
                    n185 = case shown="False" w173 {
                      selector: w173 -> [w180 w182]
                      tunnel: [cluster{u32, u32}[] [{16713728, 16713728}, {6618880, 6618880}] ("Farben [4]") cluster{u32, u32}[] [{16713728, 16713728}] ("Farben [4]")] -> w174
                      tunnel: [w180 w182] -> w176
                      frame False {
                      }
                      frame True {
                      }
                    }
                    n186 = Number To Fractional String(number=w172, precision (6)=i16 1 ("Genauigkeit (6)")) -> (F-format string=w175:string)  [unwired: 2 in]
                    n187 = global write "Global Variables.vi" "Global CCD Temperature (C)"(w172) -> ()
                    n188 = property on="CCD Status" class="Bool (strict)"("Blinking"=w176, "BoolText.Text"=w175, "Colors [4]"=w174) -> ()  [unwired: 2 in, 2 out]
                  }
                  frame #3 {
                    n189 = Tick Count (ms)() -> (millisecond timer value=w185:u32)
                    n190 = Subtract(x=w185, y=w183) -> (x-y=w184:u32)
                  }
                }
              }
            }
            "CCD Timing" <- w160
          }
          event "CCD Configure": Value Change {
            n191 = event-data() -> ("NewVal"=w187:bool)  [unwired: 1 in, 4 out]
            n192 = local read "CCD Status"() -> (w188:bool)
            n193 = And(x=w188, y=w187) -> (x .and. y?=w186:bool)
            n194 = case shown="True" w186 {
              frame False {
              }
              frame True {
                n195 = stacked-sequence {
                  frame #0 {
                    n196 = local read "Spectrum Settings"() -> (w193:T6)
                    n197 = local read "CCD Gain Number"() -> (w202:i32[])
                    n198 = local read "CCD ADC Number"() -> (w200:i32[])
                    n199 = local read "JYCCDLib.IJYCCDReqd"() -> (w191:refnum<k7>)
                    n200 = local read "CCD ADC"() -> (w199:u16)
                    n201 = local read "CCD Gain"() -> (w201:u16)
                    n202 = Unbundle By Name(w193) -> ("Integration Time"=w192:dbl)
                    n203 = local read "Image Mode"() -> (w196:bool)
                    n204 = local read "CCD Error"() -> (w195:errorcluster)
                    n205 = local read "CCD Area"() -> (w190:T1)
                    n206 = Index Array(array=w200, index=w199) -> (element=w198:i32)
                    n207 = Index Array(array=w202, index=w201) -> (element=w197:i32)
                    n208 = call "Symphony Setup.vi"("JYCCDLib.IJYCCDReqd"=w191, "ADC"=w198, "Image Mode"=w196, "Integration (s)"=w192, "Symphony Area Format"=w190, "Error Input"=w195, "Gain"=w197) -> ("DataSize"=w189:i32, "Error Output"=w194:errorcluster)  [unwired: 7 in]
                    n209 = local write "CCD Error"(w194) -> ()
                    n210 = local write "CCD Data Size"(w189) -> ()
                  }
                  frame #1 {
                    n211 = property on="Wavelength Recalculate" class="Bool (strict)"("Val(Sgnl)"=TRUE ("Value (Signaling)")) -> ()  [unwired: 2 in, 2 out]
                    n212 = local write "CCD Configure"(FALSE ("CCD Configure")) -> ()
                    n213 = local read "Image Mode"() -> (w204:bool)
                    n214 = Not(x=w204) -> (.not. x?=w203:bool)
                    n215 = property on="Spectrum" class="XYGraph (strict)"("Visible"=w203) -> ()  [unwired: 2 in, 2 out]
                    n216 = property on="Spectrum Load" class="Bool (strict)"("Visible"=w203) -> ()  [unwired: 2 in, 2 out]
                    n217 = property on="Spectrum Noise" class="DigNum (strict)"("Visible"=w203) -> ()  [unwired: 2 in, 2 out]
                    n218 = property on="CCD Current Rep." class="Str"("Visible"=w203) -> ()  [unwired: 2 in, 2 out]
                    n219 = property on="Image" class="IntGraph (strict)"("Visible"=w204) -> ()  [unwired: 2 in, 2 out]
                  }
                }
              }
            }
          }
          event Value Change {
            n220 = event-data() -> ()  [unwired: 1 in, 5 out]
            n221 = stacked-sequence {
              frame #0 {
                w220 = 1 ("y")
                n222 = local read "CCD Area"() -> (w218:T1)
                n223 = Unbundle By Name(w218) -> ("XBin"=w214:i32, "YBin"=w219:i32)
                n224 = Logarithm Base 2(1:w219) -> (0:w215:dbl)
                n225 = Logarithm Base 2(1:w214) -> (0:w211:dbl)
                n226 = Quotient & Remainder(x=w215, y=w220) -> (x-y*floor(x/y)=w216:dbl, floor(x/y)=w217:dbl)
                n227 = Quotient & Remainder(x=w211, y=w220) -> (x-y*floor(x/y)=w212:dbl, floor(x/y)=w213:dbl)
                n228 = Not Equal To 0?(x=w216) -> (x != 0?=w210:bool)
                n229 = Not Equal To 0?(x=w212) -> (x != 0?=w209:bool)
                n230 = Or(x=w209, y=w210) -> (x .or. y?=w208:bool)
                n231 = case shown="True" w210 {
                  tunnel: w217 -> [_ w225]
                  tunnel: w218 -> [_ w223]
                  frame False {
                  }
                  frame True {
                    n232 = Power Of 2(x=w225) -> (2^x=w224:dbl)
                    n233 = Bundle By Name(cluster=w223, "YBin"=w224) -> (w222:T1)
                    n234 = local write "CCD Area"(w222) -> ()
                  }
                }
                n235 = case shown="True" w209 {
                  tunnel: w213 -> [_ w229]
                  tunnel: w218 -> [_ w227]
                  frame False {
                  }
                  frame True {
                    n236 = Power Of 2(x=w229) -> (2^x=w228:dbl)
                    n237 = Bundle By Name(cluster=w227, "XBin"=w228) -> (w226:T1)
                    n238 = local write "CCD Area"(w226) -> ()
                  }
                }
                n239 = case shown="True" w208 {
                  tunnel: "Binning factor has been adjusted  (must be an exponent of 2)." ("message") -> [_ w221]
                  frame False {
                  }
                  frame True {
                    n240 = One Button Dialog(message=w221) -> ()  [unwired: 1 in, 1 out]
                  }
                }
              }
              frame #1 {
                w248 = "Could not adjust CCD area to fit binning size!" ("message")
                w249 = "CCD area has been adjusted to fit binning size." ("message")
                n241 = local read "CCD Area"() -> (w230:T1)
                n242 = Unbundle By Name(w230) -> ("XStop"=w237:i32, "XStart"=w238:i32, "XBin"=w235:i32)
                n243 = Unbundle By Name(w230) -> ("YStop"=w242:i32, "YStart"=w243:i32, "YBin"=w247:i32)
                n244 = Subtract(x=w237, y=w238) -> (x-y=w231:i32)
                n245 = Subtract(x=w242, y=w243) -> (x-y=w240:i32)
                n246 = Increment(x=w231) -> (x+1=w236:i32)
                n247 = Increment(x=w240) -> (x+1=w244:i32)
                n248 = Quotient & Remainder(x=w236, y=w235) -> (x-y*floor(x/y)=w232:i32, floor(x/y)=w234:i32)
                n249 = Quotient & Remainder(x=w244, y=w247) -> (x-y*floor(x/y)=w241:i32, floor(x/y)=w246:i32)
                n250 = Not Equal To 0?(x=w232) -> (x != 0?=w233:bool)
                n251 = Not Equal To 0?(x=w241) -> (x != 0?=w245:bool)
                n252 = case shown="True" w245 {
                  tunnel: w242 -> [_ w267]
                  tunnel: w243 -> [_ w266]
                  tunnel: w244 -> [_ w265]
                  tunnel: w246 -> [_ w264]
                  tunnel: w247 -> [_ w263]
                  tunnel: w248 -> [_ w257]
                  tunnel: w249 -> [_ w258]
                  tunnel: w230 -> [_ w262]
                  tunnel: ["" ("message") w259] -> w251
                  frame False {
                  }
                  frame True {
                    n253 = Multiply(x=w264, y=w263) -> (x*y=w269:i32)
                    n254 = Subtract(x=w265, y=w269) -> (x-y=w268:i32)
                    n255 = Add(x=w266, y=w268) -> (x+y=w261:i32)
                    n256 = Greater?(x=w267, y=w261) -> (0:w260:bool)
                    n257 = case shown="True" w260 {
                      tunnel: w262 -> [_ w274]
                      tunnel: w261 -> [_ w273]
                      tunnel: [w270 w271] -> w259
                      tunnel: w258 -> [_ w271]
                      tunnel: w257 -> [w270 _]
                      frame False {
                      }
                      frame True {
                        n258 = Bundle By Name(cluster=w274, "YStart"=w273) -> (w272:T1)
                        n259 = local write "CCD Area"(w272) -> ()
                      }
                    }
                  }
                }
                n260 = case shown="True" w233 {
                  tunnel: w234 -> [_ w289]
                  tunnel: w235 -> [_ w288]
                  tunnel: w236 -> [_ w282]
                  tunnel: w237 -> [_ w285]
                  tunnel: w238 -> [_ w283]
                  tunnel: w230 -> [_ w281]
                  tunnel: ["" ("message") w279] -> w252
                  tunnel: w249 -> [_ w278]
                  tunnel: w248 -> [_ w277]
                  frame False {
                  }
                  frame True {
                    n261 = Multiply(x=w289, y=w288) -> (x*y=w287:i32)
                    n262 = Subtract(x=w282, y=w287) -> (x-y=w284:i32)
                    n263 = Add(x=w283, y=w284) -> (x+y=w280:i32)
                    n264 = Greater?(x=w285, y=w280) -> (0:w286:bool)
                    n265 = case shown="True" w286 {
                      tunnel: w281 -> [_ w294]
                      tunnel: w280 -> [_ w292]
                      tunnel: [w290 w291] -> w279
                      tunnel: w278 -> [_ w291]
                      tunnel: w277 -> [w290 _]
                      frame False {
                      }
                      frame True {
                        n266 = Bundle By Name(cluster=w294, "XStart"=w292) -> (w293:T1)
                        n267 = local write "CCD Area"(w293) -> ()
                      }
                    }
                  }
                }
                n268 = Empty String/Path?(string/path=w252) -> (empty?=w250:bool)
                n269 = case shown="False" w250 {
                  tunnel: [w254 w255] -> w253
                  tunnel: w251 -> [_ w255]
                  tunnel: w252 -> [w254 _]
                  frame False {
                  }
                  frame True {
                  }
                }
                n270 = Empty String/Path?(string/path=w253) -> (empty?=w239:bool)
                n271 = case shown="False" w239 {
                  tunnel: w253 -> [w275 _]
                  frame False {
                    n272 = One Button Dialog(message=w275) -> ()  [unwired: 1 in, 1 out]
                  }
                  frame True {
                  }
                }
              }
            }
          }
          event "CCD Shutter": Value Change {
            n273 = event-data() -> ("NewVal"=w295:bool)  [unwired: 1 in, 4 out]
            n274 = local read "CCD Status"() -> (w296:bool)
            n275 = case shown="True" w296 {
              tunnel: w295 -> [_ w298]
              frame False {
              }
              frame True {
                n276 = local read "JYCCDLib.IJYCCDReqd"() -> (w300:refnum<k7>)
                n277 = local read "CCD Error"() -> (w299:errorcluster)
                n278 = call "Shutter Control.vi"("input error"=w299, "Shutter"=w298, "JYCCDLib.IJYCCDReqd"=w300) -> ("error out"=w301:errorcluster)  [unwired: 1 out]
                n279 = call <vilib>:"Simple Error Handler.vi"("error in (no error)"=w301) -> ("error?"=w297:bool)  [unwired: 4 in, 4 out]
                n280 = local write "CCD Error"(w301) -> ()
                n281 = case shown="True" w297 {
                  tunnel: w298 -> [_ w302]
                  frame False {
                  }
                  frame True {
                    n282 = Not(x=w302) -> (.not. x?=w303:bool)
                    n283 = local write "CCD Shutter"(w303) -> ()
                  }
                }
              }
            }
          }
          event "CCD Acquire": Value Change {
            n284 = event-data() -> ("NewVal"=w304:bool)  [unwired: 1 in, 4 out]
            n285 = case shown="True" w304 {
              frame False {
              }
              frame True {
                n286 = stacked-sequence {
                  frame #0 {
                    n287 = property on="CCD Configure" class="Bool (strict)"("Val(Sgnl)"=TRUE ("Value (Signaling)")) -> ()  [unwired: 2 in, 2 out]
                  }
                  frame #1 {
                    n288 = local read "JYCCDLib.IJYCCDReqd"() -> (w306:refnum<k7>)
                    n289 = local read "Image Mode"() -> (w310:bool)
                    n290 = local read "CCD Error"() -> (w307:errorcluster)
                    n291 = control-ref of="CCD Acquire"() -> (w308:refnum<vi>)
                    n292 = control-ref of="CCD Running"() -> (w309:refnum<vi>)
                    n293 = case shown="True" w310 {
                      tunnel: w309 -> [w314 w365]
                      tunnel: w308 -> [w313 w364]
                      tunnel: w307 -> [w312 w366]
                      tunnel: w306 -> [w311 w367]
                      frame False {
                        n294 = local read "CCD Preview"() -> (w315:bool)
                        n295 = local read "Spectrum Settings"() -> (w316:T6)
                        n296 = Unbundle By Name(w316) -> ("Repetitions"=w319:u16)
                        n297 = Select(t=i8 1, s=w315, f=w319) -> (s? t:f=w318:u16)
                        n298 = for {
                          N: w318 -> [w348]
                          tunnel: w311 -> [w340]
                          shift-right: [w353] -> _
                          shift-left: u16[][] [] -> [w354]
                          tunnel: w314 -> [w335]
                          tunnel: w313 -> [w334]
                          tunnel: w312 -> [w333]
                          i -> [w349]
                          stop <- w352 continue-if-true
                          w328 = u16 0 items=["Pixel", "Wavelength", "Energy"] ("Spectrum Axis")
                          w331 = u16 2 items=["Pixel", "Wavelength", "Energy"] ("Spectrum Axis")
                          n299 = Number To Decimal String(number=w348) -> (decimal integer string=w347:string)  [unwired: 1 in]
                          n300 = Increment(x=w349) -> (x+1=w345:i32)
                          n301 = call "Symphony Acquire Spectrum.vi"("Acquire"=w334, "Running"=w335, "Error In"=w333, "ShutterOpen"=TRUE, "JYCCDLib.IJYCCDReqd"=w340) -> ("Acq Time(ms)"=w332:u32, "Raw Data"=w338:i32[][])  [unwired: 5 in]
                          n302 = Number To Decimal String(number=w345) -> (decimal integer string=w346:string)  [unwired: 1 in]
                          n303 = local write "CCD Timing"(w332) -> ()
                          n304 = Index Array(array=w338, index (row)=0) -> (element=w336:i32[])  [unwired: 1 in]
                          n305 = Concatenate Strings(w346, "/" ("string"), w347) -> (w351:string)
                          n306 = local write "CCD Current Rep."(w351) -> ()
                          n307 = Build Array (concatenate)(w336, w354) -> (w353:i32[][])
                          n308 = local read "Wavelengths (nm)"() -> (w326:dbl[])
                          n309 = local read "Spectrum Axis"() -> (w329:u16)
                          n310 = local read "CCD Area"() -> (w325:T1)
                          n311 = call "Symphony Average Spectra.vi"("Repetitions"=w345, "Raw Spectra"=w353) -> ("Raw Spectrum"=w324:dbl[])
                          n312 = Not Equal?(x=w328, y=w329) -> (x != y?=w327:bool)
                          n313 = Equal?(x=w329, y=w331) -> (x = y?=w330:bool)
                          n314 = call "Spectrum Merge Pixels v10.5.0.vi"("CCD Area Format"=w325, "Raw Spectrum"=w324) -> ("Spectrum-Array"=w322:dbl[][])  [unwired: 1 out]
                          n315 = call "Spectrum Merge Wavelengths v10.5.0.vi"("Wavelengths (nm)"=w326, "Raw Spectrum"=w324) -> ("Spectrum-Array"=w321:dbl[][])  [unwired: 1 out]
                          n316 = local read "Spectrum Noise"() -> (w344:i64)
                          n317 = case shown="False" w327 {
                            tunnel: [w355 w356] -> w323
                            tunnel: w321 -> [_ w356]
                            tunnel: w322 -> [w355 _]
                            frame False {
                            }
                            frame True {
                            }
                          }
                          n318 = call "Spectrum Noise Subtraction v10.5.0.vi"("Spectrum Noise"=w344, "Spectrum-Array In"=w323) -> ("Spectrum-Array Out"=w343:dbl[][], "Spectrum-Cluster"=w341:T19)
                          n319 = local write "Spectrum Raw PX"(w322) -> ()
                          n320 = local write "Spectrum Raw WL"(w321) -> ()
                          n321 = case shown="False" w330 {
                            tunnel: w343 -> [_ w359]
                            tunnel: [w357 w358] -> w342
                            tunnel: w341 -> [w357 _]
                            frame False {
                            }
                            frame True {
                              n322 = call "Spectrum Jacobian Transformation v10.5.0.vi"("Spectrum-Array In"=w359) -> ("Spectrum-Cluster"=w358:T19)  [unwired: 1 in, 1 out]
                            }
                          }
                          n323 = local read "CCD Acquire"() -> (w352:bool)
                          n324 = local write "Spectrum"(w342) -> ()
                        }
                      }
                      frame True {
                        n325 = call "Symphony Acquire Image.vi"("Acquire"=w364, "Running"=w365, "Error In"=w366, "ShutterOpen"=TRUE, "JYCCDLib.IJYCCDReqd"=w367) -> ("Acq Time(ms)"=w360:u32, "Raw Data"=w363:i32[][][])  [unwired: 5 in]
                        n326 = local write "CCD Timing"(w360) -> ()
                        n327 = Index Array(array=w363, index (dim 0)=0 ("index (row)")) -> (element=w361:i32[][])  [unwired: 2 in]
                        n328 = local write "Image Raw"(w361) -> ()
                        n329 = local write "Image"(w361) -> ()
                      }
                    }
                  }
                  frame #2 {
                    n330 = local write "CCD Acquire"(FALSE ("Blinkend")) -> ()
                    n331 = local write "CCD Current Rep."("0/0" ("CCD3000 Current Rep.")) -> ()
                    n332 = local read "Spectrum Autosave"() -> (w371:bool)
                    n333 = case shown="False" w371 {
                      frame False {
                      }
                      frame True {
                        n334 = property on="Spectrum Save" class="Bool (strict)"("Val(Sgnl)"=TRUE ("Value (Signaling)")) -> ()  [unwired: 2 in, 2 out]
                      }
                    }
                  }
                }
              }
            }
          }
          event "CCD Preview": Value Change {
            n335 = event-data() -> ("NewVal"=w373:bool)  [unwired: 1 in, 4 out]
            n336 = case shown="True" w373 {
              frame False {
              }
              frame True {
                n337 = property on="CCD Acquire" class="Bool (strict)"("Val(Sgnl)"=TRUE ("Wert (signalisierend)")) -> ()  [unwired: 2 in, 2 out]
              }
            }
          }
          event "ITC Connect": Value Change {
            n338 = event-data() -> ("NewVal"=w375:bool)  [unwired: 1 in, 4 out]
            n339 = stacked-sequence {
              tunnel: w375 -> [_ w377 _]
              frame #0 {
                n340 = property on="ITC Running" class="Bool (strict)"("Blinking"=TRUE ("Blinkend")) -> ()  [unwired: 2 in, 2 out]
              }
              frame #1 {
                n341 = case shown="True" w377 {
                  selector: w377 -> [w382 _]
                  tunnel: [w382 w389] -> w379
                  frame False {
                    # "disconnect"
                    n342 = control-ref of="ITC Running"() -> (w383:refnum<vi>)
                    n343 = property class="Bool (strict)"(reference=w383, "Blinking"=w382, "Value"=w382) -> ()  [unwired: 1 in, 2 out]
                  }
                  frame True {
                    # "connect"
                    n344 = local read "ITC Selector"() -> (w390:u16)
                    n345 = call "ITC503 Connect.vi"("ITC Selector"=w390) -> ("ITC Setup"=w388:T12, "Connected"=w389:bool)
                    n346 = local write "ITC Setup"(w388) -> ()
                    n347 = call "ITC503 Get Values.vi"("ITC Setup"=w388) -> ("ITC503 Current Values"=w387:T2)  [unwired: 1 in, 1 out]
                    n348 = Unbundle By Name(w387) -> ("ITC503 Setpoint"=w384:dbl)
                    n349 = Bundle By Name(cluster=T3 {"ITC503 Set Setpoint"=0.0, "ITC503 Set Auto Heater"=TRUE, "ITC503 Set Auto PID"=TRUE, "P"=0.0, "I"=0.0, "D"=0.0} ("ITC503 Settings"), "ITC503 Set Setpoint"=w384) -> (w385:T3)
                    n350 = local write "ITC Settings"(w385) -> ()
                  }
                }
                n351 = case shown="False" w379 {
                  tunnel: [T16."Disabled and Grayed Out" ("Deaktiviert") T16."Enabled" ("Deaktiviert")] -> w378
                  frame False {
                  }
                  frame True {
                  }
                }
                n352 = local write "ITC Status"(w379) -> ()
                n353 = local write "ITC Connect"(w379) -> ()
                n354 = property on="ITC Configure" class="Bool (strict)"("DisabledEnum"=w378) -> ()  [unwired: 2 in, 2 out]
              }
              frame #2 {
                n355 = property on="ITC Running" class="Bool (strict)"("Blinking"=FALSE ("Blinkend")) -> ()  [unwired: 2 in, 2 out]
                n356 = property on="ITC Read" class="Bool (strict)"("Val(Sgnl)"=TRUE ("Wert (signalisierend)")) -> ()  [unwired: 2 in, 2 out]
              }
            }
          }
          event "ITC Read": Value Change {
            n357 = event-data() -> ("Time"=w394:u32, "NewVal"=w398:bool)  [unwired: 1 in, 3 out]
            n358 = local read "ITC Status"() -> (w397:bool)
            n359 = control-ref of="ITC Running"() -> (w395:refnum<vi>)
            n360 = And(x=w397, y=w398) -> (x .and. y?=w396:bool)
            n361 = case shown="True" w396 {
              tunnel: w395 -> [w400 w404]
              tunnel: w394 -> [_ w403]
              tunnel: [u32 0 w402] -> w393
              frame False {
                n362 = property class="Bool (strict)"(reference=w400, "BoolText.Text"="" ("Boolescher Text.Text")) -> ()  [unwired: 1 in, 2 out]
              }
              frame True {
                n363 = stacked-sequence {
                  seq-local: [_ w410 _ _] -> [_ _ w426 _]
                  seq-local: [w405 _ _ _] -> [_ _ _ w432]
                  tunnel: w404 -> [_ _ w419 _]
                  tunnel: w403 -> [_ w411 _ _]
                  tunnel: [_ _ _ w433] -> w402
                  frame #0 {
                    n364 = Tick Count (ms)() -> (millisecond timer value=w405:u32)
                  }
                  frame #1 {
                    n365 = local read "ITC Setup"() -> (w417:T12)
                    n366 = local read "ITC Gradient Time"() -> (w415:i64)
                    n367 = call "ITC503 Get Values.vi"("ITC Setup"=w417) -> ("ITC503 Current Values"=w410:T2)  [unwired: 1 in, 1 out]
                    n368 = local read "ITC Temp Storage"() -> (w409:dbl)
                    n369 = Unbundle By Name(w410) -> ("ITC503 Temperature"=w407:dbl)
                    n370 = Subtract(x=w411, y=w415) -> (x-y=w414:i64)
                    n371 = Divide(x=w414, y=i64 1000) -> (x/y=w412:dbl)
                    n372 = Subtract(x=w407, y=w409) -> (x-y=w408:dbl)
                    n373 = Divide(x=w408, y=w412) -> (x/y=w416:dbl)
                    n374 = Bundle By Name(cluster=w410, "ITC503 Gradient"=w416) -> (w406:T2)
                    n375 = local write "ITC Current Values"(w406) -> ()
                    n376 = global write "Global Variables.vi" "Global ITC Values"(w406) -> ()
                  }
                  frame #2 {
                    n377 = Unbundle By Name(w426) -> ("ITC503 Temperature"=w418:dbl, "ITC503 Setpoint"=w427:dbl)
                    n378 = Subtract(x=w418, y=w427) -> (x-y=w428:dbl)
                    n379 = Number To Fractional String(number=w418, precision (6)=i16 2 ("Genauigkeit (6)")) -> (F-format string=w422:string)  [unwired: 2 in]
                    n380 = Absolute Value(x=w428) -> (abs(x)=w429:dbl)
                    n381 = String Subset(string=w422, length (rest)=5 ("Länge (Rest)")) -> (substring=w420:string)  [unwired: 1 in]
                    n382 = Greater?(x=w429, y=2.0) -> (0:w425:bool)
                    n383 = Not(x=w425) -> (.not. x?=w424:bool)
                    n384 = property class="Bool (strict)"(reference=w419, "Blinking"=w425, "Value"=w424, "BoolText.Text"=w420) -> ()  [unwired: 1 in, 2 out]
                    n385 = local write "ITC Temp Storage"(w418) -> ()
                  }
                  frame #3 {
                    n386 = Tick Count (ms)() -> (millisecond timer value=w431:u32)
                    n387 = local write "ITC Gradient Time"(w431) -> ()
                    n388 = Subtract(x=w431, y=w432) -> (x-y=w433:u32)
                  }
                }
              }
            }
            n389 = local write "ITC Timing"(w393) -> ()
          }
          event "ITC Configure": Value Change {
            n390 = event-data() -> ("NewVal"=w434:bool)  [unwired: 1 in, 4 out]
            n391 = stacked-sequence {
              tunnel: w434 -> [_ w436 _]
              frame #0 {
                n392 = property on="ITC Running" class="Bool (strict)"("Blinking"=TRUE ("Blinkend")) -> ()  [unwired: 2 in, 2 out]
              }
              frame #1 {
                n393 = local read "ITC Status"() -> (w438:bool)
                n394 = And(x=w438, y=w436) -> (x .and. y?=w437:bool)
                n395 = case shown="True" w437 {
                  frame False {
                  }
                  frame True {
                    n396 = local read "ITC Settings"() -> (w439:T3)
                    n397 = local read "ITC Setup"() -> (w440:T12)
                    n398 = call "ITC503 Set Values.vi"("Set Channel"=i16 1, "ITC503 Settings"=w439, "ITC Setup"=w440) -> ()  [unwired: 2 in]
                  }
                }
              }
              frame #2 {
                w443 = FALSE ("Blinkend")
                n399 = property on="ITC Running" class="Bool (strict)"("Blinking"=w443) -> ()  [unwired: 2 in, 2 out]
                n400 = local write "ITC Configure"(w443) -> ()
                n401 = property on="ITC Read" class="Bool (strict)"("Val(Sgnl)"=TRUE ("Wert (signalisierend)")) -> ()  [unwired: 2 in, 2 out]
              }
            }
          }
          event "Drive Connect": Value Change {
            n402 = event-data() -> ("NewVal"=w444:bool)  [unwired: 1 in, 4 out]
            n403 = stacked-sequence {
              tunnel: w444 -> [_ w448 _ _]
              frame #0 {
                n404 = property on="Drive Running" class="Bool (strict)"("Blinking"=TRUE ("Blinkend")) -> ()  [unwired: 2 in, 2 out]
              }
              frame #1 {
                n405 = local read "Drive Connection"() -> (w449:T5)
                n406 = Not(x=w448) -> (.not. x?=w450:bool)
                n407 = call "ESA-C Connect.vi"("Remote=F /Local=T"=w450, "Drive Connection Settings"=w449) -> ("Success"=w451:bool)  [unwired: 2 in]
                n408 = Exclusive Or(1:w450, 2:w451) -> (0:w452:bool)
                n409 = local write "Drive Connect"(w452) -> ()
                n410 = local write "Drive Status"(w452) -> ()
                n411 = case shown="False" w452 {
                  tunnel: [T16."Disabled and Grayed Out" ("Deaktiviert") T16."Enabled" ("Deaktiviert")] -> w447
                  tunnel: ["" ("Boolescher Text.Text") w455] -> w446
                  frame False {
                  }
                  frame True {
                    n412 = property on="Drive Selector" class="Ring (strict)"() -> ("RingText.Text"=w455:string)  [unwired: 2 in, 2 out]
                  }
                }
                n413 = property on="Drive Live Controls" class="Clust (strict)"("DisabledEnum"=w447) -> ()  [unwired: 2 in, 2 out]
                n414 = property on="Drive Status" class="Bool (strict)"("BoolText.Text"=w446) -> ()  [unwired: 2 in, 2 out]
                n415 = property on="Drive GoTo" class="Bool (strict)"("DisabledEnum"=w447) -> ()  [unwired: 2 in, 2 out]
              }
              frame #2 {
                # "prepare mirroring values to target controls"
                n416 = local write "Drive Copy Target"(TRUE ("Copy Drive Target")) -> ()
              }
              frame #3 {
                n417 = property on="Drive Running" class="Bool (strict)"("Blinking"=FALSE ("Blinkend")) -> ()  [unwired: 2 in, 2 out]
                n418 = property on="Drive Read" class="Bool (strict)"("Val(Sgnl)"=TRUE ("Wert (signalisierend)")) -> ()  [unwired: 2 in, 2 out]
              }
            }
          }
          event "Drive Read": Value Change {
            n419 = event-data() -> ("NewVal"=w463:bool)  [unwired: 1 in, 4 out]
            n420 = local read "Drive Status"() -> (w462:bool)
            n421 = And(x=w462, y=w463) -> (x .and. y?=w461:bool)
            n422 = case shown="True" w461 {
              tunnel: [u32 0 w465] -> w460
              frame False {
              }
              frame True {
                n423 = stacked-sequence {
                  seq-local: [w466 _ _ _] -> [_ _ _ w472]
                  tunnel: [_ _ _ w471] -> w465
                  frame #0 {
                    n424 = Tick Count (ms)() -> (millisecond timer value=w466:u32)
                  }
                  frame #1 {
                    n425 = local read "Drive Connection"() -> (w468:T5)
                    n426 = call "ESA-C Get Values.vi"("Drive Connection Settings"=w468) -> ("Drive Current Values"=w467:T4)
                    n427 = local write "Drive Live Current Values"(w467) -> ()
                    n428 = local write "Drive Current Values"(w467) -> ()
                    n429 = global write "Global Variables.vi" "Global Drive Position"(w467) -> ()
                  }
                  frame #2 {
                    n430 = local read "Drive Copy Target"() -> (w469:bool)
                    n431 = case shown="True" w469 {
                      frame False {
                      }
                      frame True {
                        n432 = property on="Drive Copy Target" class="Bool (strict)"("Val(Sgnl)"=TRUE ("Value (Signaling)")) -> ()  [unwired: 2 in, 2 out]
                      }
                    }
                  }
                  frame #3 {
                    n433 = Tick Count (ms)() -> (millisecond timer value=w473:u32)
                    n434 = Subtract(x=w473, y=w472) -> (x-y=w471:u32)
                  }
                }
              }
            }
            "Drive Timing" <- w460
          }
          event "Drive GoTo": Value Change {
            n435 = event-data() -> ("NewVal"=w474:bool)  [unwired: 1 in, 4 out]
            n436 = stacked-sequence {
              tunnel: w474 -> [_ w476 _]
              frame #0 {
                n437 = property on="Drive Running" class="Bool (strict)"("Blinking"=TRUE ("Blinkend")) -> ()  [unwired: 2 in, 2 out]
              }
              frame #1 {
                n438 = local read "Drive Status"() -> (w478:bool)
                n439 = And(x=w478, y=w476) -> (x .and. y?=w477:bool)
                n440 = case shown="True" w477 {
                  frame False {
                  }
                  frame True {
                    n441 = local read "Drive New Positions"() -> (w479:T7)
                    n442 = local read "Drive Connection"() -> (w480:T5)
                    n443 = control-ref of="Drive Running"() -> (w481:refnum<vi>)
                    n444 = call "ESA-C Move Absolute.vi"("Running"=w481, "Drive New Abs. Positions"=w479, "Drive Connection Settings"=w480) -> ()  [unwired: 2 in]
                  }
                }
              }
              frame #2 {
                w483 = FALSE ("Blinkend")
                n445 = local write "Drive GoTo"(w483) -> ()
                n446 = property on="Drive Running" class="Bool (strict)"("Blinking"=w483) -> ()  [unwired: 2 in, 2 out]
                n447 = property on="Drive Read" class="Bool (strict)"("Val(Sgnl)"=TRUE ("Wert (signalisierend)")) -> ()  [unwired: 2 in, 2 out]
              }
            }
          }
          event Value Change {
            n448 = event-data() -> ("NewVal"=w485:bool)  [unwired: 1 in, 4 out]
            n449 = local read "Drive Status"() -> (w486:bool)
            n450 = And(x=w486, y=w485) -> (x .and. y?=w484:bool)
            n451 = case shown="True" w484 {
              frame False {
              }
              frame True {
                n452 = stacked-sequence {
                  seq-local: [w487 _ _] -> [_ _ _]
                  frame #0 {
                    # "Move and Read"
                    n453 = flat-sequence {
                      tunnel: [w494] -> w490
                      tunnel: [w491] -> w489
                      tunnel: w490 -> [w496]
                      tunnel: w489 -> [w497]
                      tunnel: [w495] -> w488
                      tunnel: w488 -> [w502]
                      tunnel: [w502] -> w487
                      frame #0 {
                        n454 = local read "Drive Live Controls"() -> (w491:T10)
                        n455 = local read "Drive Connection"() -> (w492:T5)
                        n456 = control-ref of="Drive Running"() -> (w493:refnum<vi>)
                        n457 = call "ESA-C Live Control v10.4.0.vi"("Running"=w493, "Drive Live Controls"=w491, "Drive Connection Settings"=w492) -> ("Reset Switches"=w494:bool)  [unwired: 1 in]
                      }
                      frame #1 {
                        n458 = case shown="True" w496 {
                          tunnel: w497 -> [w498 w501]
                          tunnel: [w498 w500] -> w495
                          frame False {
                          }
                          frame True {
                            w499 = FALSE ("Move Out")
                            n459 = Bundle By Name(cluster=w501, "Move Home"=w499, "Move Down"=w499, "Move Up"=w499, "Move Left"=w499, "Move Right"=w499, "Move Out"=w499, "Move In"=w499) -> (w500:T10)
                          }
                        }
                      }
                      frame #2 {
                        n460 = local write "Drive Live Controls"(w502) -> ()
                      }
                    }
                  }
                  frame #1 {
                    n461 = local write "Drive Copy Target"(TRUE ("Copy Drive Target")) -> ()
                  }
                  frame #2 {
                    n462 = property on="Drive Read" class="Bool (strict)"("Val(Sgnl)"=TRUE ("Wert (signalisierend)")) -> ()  [unwired: 2 in, 2 out]
                  }
                }
              }
            }
          }
          event "Drive Copy Target": Value Change {
            # "this event is triggered after drive readout\nit should usually not be triggered directly by signaling"
            n463 = event-data() -> ("NewVal"=w505:bool)  [unwired: 1 in, 4 out]
            n464 = case shown="True" w505 {
              frame False {
              }
              frame True {
                n465 = stacked-sequence {
                  frame #0 {
                    n466 = local read "Drive Current Values"() -> (w507:T4)
                    n467 = Unbundle By Name(w507) -> ("Position"=w506:T20)
                    n468 = local write "Drive New Positions"(w506) -> ()
                  }
                  frame #1 {
                    n469 = local write "Drive Copy Target"(FALSE ("Copy Drive Target")) -> ()
                  }
                }
              }
            }
          }
          event "Wavelength Recalculate": Value Change {
            n470 = event-data() -> ("NewVal"=w509:bool)  [unwired: 1 in, 4 out]
            n471 = case shown="True" w509 {
              frame False {
              }
              frame True {
                n472 = local read "Mono Current Values"() -> (w512:T9)
                n473 = local read "CCD Area"() -> (w510:T1)
                n474 = call "iHR550 Convert Axis v10.5.0.vi"("CCD Area Format"=w510, "iHR Current Values"=w512) -> ("Wavelengths (nm)"=w511:dbl[])
                n475 = local write "Wavelengths (nm)"(w511) -> ()
                n476 = global write "Global Variables.vi" "Global Wavelengths (nm)"(w511) -> ()
              }
            }
          }
          event Value Change {
            n477 = event-data() -> ()  [unwired: 1 in, 5 out]
            n478 = property on="CCD Configure" class="Bool (strict)"("Val(Sgnl)"=TRUE ("Value (Signaling)")) -> ()  [unwired: 2 in, 2 out]
          }
          event "Spectrum Axis": Value Change {
            w526 = u16 2 items=["Pixel", "Wavelength", "Energy"] ("Spectrum Axis")
            w528 = u16 0 items=["Pixel", "Wavelength", "Energy"] ("Spectrum Axis")
            n479 = event-data() -> ("NewVal"=w524:u16)  [unwired: 1 in, 4 out]
            n480 = Equal?(x=w524, y=w528) -> (x = y?=w527:bool)
            n481 = case shown="False" w527 {
              tunnel: [w546 w548] -> w525
              tunnel: [w545 w547] -> w520
              tunnel: "Pixel" ("X Scale.Name Label.Text") -> [_ w547]
              tunnel: "Wavelength (nm)" ("X Scale.Name Label.Text") -> [w545 _]
              frame False {
                n482 = local read "Spectrum Raw WL"() -> (w546:dbl[][])
              }
              frame True {
                n483 = local read "Spectrum Raw PX"() -> (w548:dbl[][])
              }
            }
            n484 = local read "Spectrum Noise"() -> (w515:i64)
            n485 = Equal?(x=w524, y=w526) -> (x = y?=w523:bool)
            n486 = call "Spectrum Noise Subtraction v10.5.0.vi"("Spectrum Noise"=w515, "Spectrum-Array In"=w525) -> ("Spectrum-Array Out"=w522:dbl[][], "Spectrum-Cluster"=w514:T19)
            n487 = case shown="True" w523 {
              tunnel: w522 -> [_ w536]
              tunnel: [w530 w535] -> w521
              tunnel: w514 -> [w530 w534]
              tunnel: w520 -> [w529 w531]
              tunnel: [w529 w533] -> w517
              tunnel: "Energy (eV)" ("X Scale.Name Label.Text") -> [_ w532]
              tunnel: w515 -> [_ w537]
              frame False {
              }
              frame True {
                # "Jacobian Transformation requires noise subtraction"
                n488 = Greater Than 0?(x=w537) -> (x > 0?=w538:bool)
                n489 = case shown="False" w538 {
                  tunnel: w536 -> [_ w544]
                  tunnel: [w540 w543] -> w535
                  tunnel: w534 -> [w540 _]
                  tunnel: [w539 w542] -> w533
                  tunnel: w532 -> [_ w542]
                  tunnel: w531 -> [w539 _]
                  frame False {
                    w541 = u16 1 items=["Pixel", "Wavelength", "Energy"] ("Spectrum Axis")
                    n490 = call "Display Message to User"() -> ()  [unwired: 10 in, 2 out]
                    n491 = local write "Spectrum Axis"(w541) -> ()
                  }
                  frame True {
                    n492 = call "Spectrum Jacobian Transformation v10.5.0.vi"("Spectrum-Array In"=w544) -> ("Spectrum-Cluster"=w543:T19)  [unwired: 1 in, 1 out]
                  }
                }
              }
            }
            n493 = local write "Spectrum"(w521) -> ()
            n494 = property on="Spectrum" class="XYGraph (strict)"("XScale.NameLbl.Text"=w517) -> ()  [unwired: 2 in, 2 out]
          }
          event "Spectrum Noise": Value Change {
            n495 = event-data() -> ("NewVal"=w551:i64)  [unwired: 1 in, 4 out]
            n496 = Greater Than 0?(x=w551) -> (x > 0?=w550:bool)
            n497 = case shown="True" w550 {
              tunnel: [w552 w553] -> w549
              frame False {
                w552 = u16 1 items=["Pixel", "Wavelength", "Energy"] ("Spectrum Axis")
                # "Disable Jacobian Transformation"
              }
              frame True {
                n498 = local read "Spectrum Axis"() -> (w553:u16)
              }
            }
            n499 = property on="Spectrum Axis" class="Ring (strict)"("Val(Sgnl)"=w549) -> ()  [unwired: 2 in, 2 out]
          }
          event "Spectrum Save": Value Change {
            n500 = event-data() -> ("NewVal"=w554:bool)  [unwired: 1 in, 4 out]
            n501 = stacked-sequence {
              tunnel: w554 -> [w555 _]
              frame #0 {
                n502 = case shown="True" w555 {
                  frame False {
                  }
                  frame True {
                    n503 = local read "Mono Current Values"() -> (w566:T9)
                    n504 = local read "Drive Current Values"() -> (w564:T4)
                    n505 = local read "ITC Current Values"() -> (w563:T2)
                    n506 = local read "CCD Temperature"() -> (w562:dbl)
                    n507 = local read "Spectrum Settings"() -> (w565:T6)
                    n508 = local read "Image Mode"() -> (w561:bool)
                    n509 = case shown="True" w561 {
                      tunnel: w566 -> [w571 w585]
                      tunnel: w565 -> [w572 w584]
                      tunnel: w564 -> [w573 w583]
                      tunnel: w563 -> [w570 w582]
                      tunnel: w562 -> [w574 w581]
                      tunnel: [w569 w579] -> w558
                      tunnel: ["Spectrum" ("Export Type") "Image" ("Export Type")] -> w557
                      tunnel: [w567 w577] -> w556
                      frame False {
                        n510 = local read "Spectrum Raw WL"() -> (w567:dbl[][])
                        n511 = call "Export_spectrumFileName.vi"("ITC503 Current Values"=w570, "iHR Current Values"=w571, "Spectra Settings"=w572, "Drive Current Values"=w573, "CCD3500 Temperature"=w574) -> ("Filename"=w569:string)
                      }
                      frame True {
                        n512 = local read "Image Raw"() -> (w576:i32[][])
                        n513 = local read "CCD Area"() -> (w578:T1)
                        n514 = call "Export_imageFileName.vi"("ITC503 Current Values"=w582, "iHR Current Values"=w585, "Spectra Settings"=w584, "Drive Current Values"=w583, "CCD3500 Temperature"=w581) -> ("Filename"=w579:string)
                        n515 = Transpose 2D Array(2D array=w576) -> (transposed array=w575:i32[][])
                        n516 = call "Image Merge Axes.vi"("Image In"=w575, "CCD Area Format"=w578) -> ("Image Out"=w577:dbl[][])  [unwired: 13 in]
                      }
                    }
                    n517 = local read "Spectrum Autosave"() -> (w559:bool)
                    n518 = local read "Auto Folder"() -> (w560:path)
                    n519 = call "Export_2DtoTxt v10.2.0.vi"("Auto Folder"=w560, "Auto?"=w559, "Data (2D)"=w556, "Export Type"=w557, "Filename"=w558) -> ()  [unwired: 1 in]
                  }
                }
              }
              frame #1 {
                n520 = local write "Spectrum Save"(FALSE ("Spectrum Save")) -> ()
              }
            }
          }
          event "Spectrum Load": Value Change {
            n521 = event-data() -> ("NewVal"=w587:bool)  [unwired: 1 in, 4 out]
            n522 = case shown="True" w587 {
              frame False {
              }
              frame True {
                n523 = stacked-sequence {
                  seq-local: [w588 _ _] -> [_ w591 _]
                  frame #0 {
                    n524 = call "Load Spectrum.vi"() -> ("Intensity"=w588:dbl[], "Wavelength"=w590:dbl[])  [unwired: 3 in, 1 out]
                    n525 = Build Array(w590, w588) -> (w589:dbl[][])
                    n526 = local write "Spectrum Raw WL"(w589) -> ()
                  }
                  frame #1 {
                    n527 = call <vilib>:"Median.vi"("X"=w591) -> ("median"=w593:dbl)  [unwired: 1 out]
                    n528 = To Long Integer(number=w593) -> (32bit integer=w592:i32)
                    n529 = property on="Spectrum Noise" class="DigNum (strict)"("Val(Sgnl)"=w592) -> ()  [unwired: 2 in, 2 out]
                  }
                  frame #2 {
                    n530 = local write "Spectrum Load"(FALSE ("Spectrum Load")) -> ()
                  }
                }
              }
            }
          }
          event "Spectrum Autosave": Value Change {
            n531 = event-data() -> ("NewVal"=w596:bool)  [unwired: 1 in, 4 out]
            n532 = case shown="True" w596 {
              tunnel: [path "" w602] -> w595
              frame False {
              }
              frame True {
                n533 = call "File Dialog"("prompt"="Choose Save Folder") -> ("selected path"=w604:path, "cancelled"=w598:bool, "error out"=w600:errorcluster)  [unwired: 11 in, 1 out]
                n534 = call <vilib>:"Simple Error Handler.vi"("error in (no error)"=w600) -> ("error?"=w599:bool)  [unwired: 4 in, 4 out]
                n535 = Or(x=w598, y=w599) -> (x .or. y?=w601:bool)
                n536 = case shown="True" w601 {
                  tunnel: w604 -> [w605 _]
                  tunnel: [w605 path ""] -> w602
                  frame False {
                  }
                  frame True {
                    n537 = local write "Spectrum Autosave"(FALSE ("Spectrum Autosave")) -> ()
                  }
                }
              }
            }
            n538 = local write "Auto Folder"(w595) -> ()
          }
          event "Spectrum Maximize": Value Change {
            # "Currently disabled by hiding control!"
            n539 = event-data() -> ("NewVal"=w608:bool)  [unwired: 1 in, 4 out]
            n540 = case shown="True" w608 {
              frame False {
                n541 = local read "Spectrum Properties"() -> (w611:cluster{"Position":T11, "Plot Area Size":T11})
                n542 = Unbundle(w611) -> ("Position"=w610:T11, "Plot Area Size"=w609:T11)
                n543 = stacked-sequence {
                  tunnel: w610 -> [_ w613]
                  tunnel: w609 -> [w612 _]
                  frame #0 {
                    n544 = property on="Spectrum" class="XYGraph (strict)"("Plot Area Size"=w612) -> ()  [unwired: 2 in, 2 out]
                  }
                  frame #1 {
                    n545 = property on="Spectrum" class="XYGraph (strict)"("Position"=w613) -> ()  [unwired: 2 in, 2 out]
                  }
                }
              }
              frame True {
                n546 = property on="Spectrum" class="XYGraph (strict)"() -> ("Bounds"=w634:T11, "Plot Area Size"=w633:T11, "Position"=w631:T21)  [unwired: 2 in, 2 out]
                n547 = Bundle("Position"=w631, "Plot Area Size"=w633) -> (w632:cluster{"Position":T21, "Plot Area Size":T11})  [unwired: 1 in]
                n548 = Unbundle By Name(w634) -> ("Width"=w638:u32, "Height"=w639:u32)
                n549 = Unbundle By Name(w633) -> ("Width"=w641:u32, "Height"=w640:u32)
                n550 = property on="Register" class="TabCtl (strict)"() -> ("Bounds"=w637:T11, "Position"=w626:T21, "Width"=w617:u32, "Height"=w616:u32)  [unwired: 2 in, 2 out]
                n551 = local write "Spectrum Properties"(w632) -> ()
                n552 = Subtract(x=w638, y=w641) -> (x-y=w630:u32)
                n553 = Subtract(x=w639, y=w640) -> (x-y=w627:u32)
                n554 = Add(x=w630, y=u32 25) -> (x+y=w629:u32)
                n555 = Add(x=w627, y=u32 70) -> (x+y=w628:u32)
                n556 = Subtract(x=w617, y=w629) -> (x-y=w636:u32)
                n557 = Subtract(x=w616, y=w628) -> (x-y=w635:u32)
                n558 = Bundle By Name(cluster=w637, "Width"=w636, "Height"=w635) -> (w614:T11)
                n559 = Unbundle By Name(w626) -> ("Left"=w625:i32, "Top"=w622:i32)
                n560 = Add(x=w625, y=20) -> (x+y=w624:i32)
                n561 = Add(x=w622, y=50) -> (x+y=w623:i32)
                n562 = Bundle By Name(cluster=w626, "Left"=w624, "Top"=w623) -> (w615:T21)
                n563 = stacked-sequence {
                  tunnel: w615 -> [w642 _]
                  tunnel: w614 -> [_ w643]
                  frame #0 {
                    n564 = property on="Spectrum" class="XYGraph (strict)"("Position"=w642) -> ()  [unwired: 2 in, 2 out]
                  }
                  frame #1 {
                    n565 = property on="Spectrum" class="XYGraph (strict)"("Plot Area Size"=w643) -> ()  [unwired: 2 in, 2 out]
                  }
                }
              }
            }
          }
          event "Mapping Start": Value Change {
            n566 = event-data() -> ("NewVal"=w644:bool)  [unwired: 1 in, 4 out]
            n567 = case shown="True" w644 {
              frame False {
              }
              frame True {
                n568 = local read "JYCCDLib.IJYCCDReqd"() -> (w680:refnum<k7>)
                n569 = local read "Drive Current Values"() -> (w675:T4)
                n570 = local read "ITC Current Values"() -> (w677:T2)
                n571 = local read "Mono Current Values"() -> (w676:T9)
                n572 = local read "CCD Temperature"() -> (w682:dbl)
                n573 = vi-ref "Mapping v10.5.0.vi"() -> (w662:refnum<vi>)
                n574 = local read "Wavelengths (nm)"() -> (w678:dbl[])
                n575 = local read "Drive Status"() -> (w673:bool)
                n576 = local read "Drive Connection"() -> (w679:T5)
                n577 = local read "Spectrum Settings"() -> (w681:T6)
                n578 = local read "CCD Status"() -> (w671:bool)
                n579 = local read "CCD Status"() -> (w655:bool)
                n580 = Not(x=w673) -> (.not. x?=w672:bool)
                n581 = Not(x=w671) -> (.not. x?=w670:bool)
                n582 = Not(x=w655) -> (.not. x?=w654:bool)
                n583 = Bundle By Name(cluster=T18 {"Drive Connection Settings"={"Objective GPIB-Port"=1, "Stage GPIB-Port"=0, "Drive Selector"=5, "Drive Velocity (V/s)"=1.0}, "ITC503 Current Values"={"ITC503 Heater"=4.0, "ITC503 Temperature"=4.0, "ITC503 P"=0.0, "ITC503 I"=5.0, "ITC503 D"=0.0, "ITC503 Setpoint"=0.0, "ITC503 Gradient"=0.0, "ITC503 Heater Auto"=FALSE, "ITC503 PID Auto"=FALSE}, "Wavelengths (nm)"=[], "Drive Current Values"={"Voltages"={"Drive X Voltage"=0.0, "Drive Y Voltage"=0.0, "Drive Z Voltage"=0.0}, "Position"={"Drive X Position"=0.0, "Drive Y Position"=0.0, "Drive Z Position"=0.0}}, "iHR Current Values"={"iHR 550 Front Entrance"=0.0, "iHR550 Side Exit"=0.0, "iHR550 Wavelength"=897.9988, "iHR550 Exit Mirror"=2, "iHR550 Grating"="1", "Grating Index"=1}, "Spectra Settings"={"Integration Time"=0.0, "Repetitions"=0, "Mapping Spectra"=TRUE}, "CCD3500 Temperature"=0.0, "Simulate Drive"=FALSE, "Simulate Spectra"=FALSE, "JYCCDLib.IJYCCDReqd"=refnum} ("Input Parameters"), "JYCCDLib.IJYCCDReqd"=w680, "Drive Connection Settings"=w679, "ITC503 Current Values"=w677, "Wavelengths (nm)"=w678, "Drive Current Values"=w675, "iHR Current Values"=w676, "Spectra Settings"=w681, "CCD3500 Temperature"=w682, "Simulate Drive"=w672, "Simulate Spectra"=w670) -> (w663:T18)
                n584 = invoke class="VI" method="Ctrl Val.Set"(reference=w662, "Control Name"="Simulate Spectra", "Value"=w654) -> (reference out=w661:refnum<vi>, error out=w656:errorcluster)  [unwired: 2 in, 3 out]
                n585 = local read "Drive Status"() -> (w653:bool)
                n586 = Not(x=w653) -> (.not. x?=w652:bool)
                n587 = invoke class="VI" method="Ctrl Val.Set"(reference=w661, error in=w656, "Control Name"="Simulate Drive", "Value"=w652) -> (reference out=w660:refnum<vi>, error out=w657:errorcluster)  [unwired: 1 in, 3 out]
                n588 = invoke class="VI" method="Ctrl Val.Set"(reference=w660, error in=w657, "Control Name"="Input Parameters", "Value"=w663) -> (reference out=w650:refnum<vi>, error out=w647:errorcluster)  [unwired: 1 in, 3 out]
                n589 = property on="Measurement Running" class="Bool (strict)"("Blinking"=TRUE ("Blinkend")) -> ()  [unwired: 2 in, 2 out]
                n590 = invoke class="VI" method="Ctrl Val.Set"(reference=w650, error in=w647, "Control Name"="AutoClose", "Value"=TRUE ("Blinkend")) -> (reference out=w649:refnum<vi>, error out=w648:errorcluster)  [unwired: 1 in, 3 out]
                n591 = invoke on="Invoke Node" class="VI" method="FP.Open"(reference=w649, error in=w648, "Activate"=TRUE ("Activate?")) -> (reference out=w665:refnum<vi>, error out=w664:errorcluster)  [unwired: 2 in, 3 out]
                n592 = invoke on="Invoke Node" class="VI" method="Run VI"(reference=w665, error in=w664, "Wait until done"=FALSE ("Wait Until Done"), "Auto Dispose Ref"=TRUE ("Auto Dispose Reference")) -> ()  [unwired: 1 in, 5 out]
              }
            }
          }
          event "Video Show": Value Change {
            n593 = event-data() -> ("NewVal"=w683:bool)  [unwired: 1 in, 4 out]
            n594 = case shown="True" w683 {
              frame False {
              }
              frame True {
                w684 = "true" ("Control Name")
                n595 = vi-ref "Video Toolset v10.0.0.vi"() -> (w700:refnum<vi>)
                n596 = invoke class="VI" method="Ctrl Val.Set"(reference=w700, "Control Name"="AutorunText", "Value"=w684) -> (reference out=w689:refnum<vi>, error out=w688:errorcluster)  [unwired: 2 in, 3 out]
                n597 = invoke class="VI" method="Ctrl Val.Set"(reference=w689, error in=w688, "Control Name"="AutocloseText", "Value"=w684) -> (reference out=w685:refnum<vi>, error out=w686:errorcluster)  [unwired: 1 in, 3 out]
                n598 = local read "Camera Name"() -> (w692:string)
                n599 = local read "Snapshot Folder"() -> (w691:path)
                n600 = invoke class="VI" method="Ctrl Val.Set"(reference=w685, error in=w686, "Control Name"="Source Name", "Value"=w692) -> (reference out=w697:refnum<vi>, error out=w696:errorcluster)  [unwired: 1 in, 3 out]
                n601 = invoke class="VI" method="Ctrl Val.Set"(reference=w697, error in=w696, "Control Name"="Capture Folder", "Value"=w691) -> (reference out=w698:refnum<vi>, error out=w699:errorcluster)  [unwired: 1 in, 3 out]
                n602 = invoke on="Invoke Node" class="VI" method="FP.Open"(reference=w698, error in=w699, "Activate"=TRUE ("Activate?")) -> (reference out=w702:refnum<vi>, error out=w701:errorcluster)  [unwired: 2 in, 3 out]
                n603 = local write "Video Show"(FALSE ("Video Show")) -> ()
                n604 = invoke on="Invoke Node" class="VI" method="Run VI"(reference=w702, error in=w701, "Wait until done"=FALSE ("Wait Until Done"), "Auto Dispose Ref"=TRUE ("Auto Dispose Reference")) -> ()  [unwired: 1 in, 5 out]
              }
            }
          }
        }
      }
    }
    frame #3 {
      # "Close Connections"
      n605 = control-ref of="Dieses VI"() -> (w706:refnum<vi>)
      n606 = invoke class="VI" method="Default Vals.Reinit All"(reference=w706) -> ()  [unwired: 2 in, 3 out]
    }
  }
